vi "OOB Performance Test.vi"() -> ()   [LabVIEW 2021]
uses:
  <vilib>/Platform/TimedLoop/XDataNode/timing_clust.ctl
  <vilib>/Platform/TimedLoop/XDataNode/nitl_modes.ctl
  <vilib>/Platform/TimedLoop/XDataNode/wakeup.ctl
  CIFOutOfBand.lvclass/CIFOutOfBand.ctl
  CIFOutOfBand.lvclass
  <vilib>/Platform/TimedLoop/XDataNode/XDataNode.xnode
  <vilib>/Platform/TimedLoop/XDataNode/XDNodeRunTimeDep.lvlib
panel:
  out "avg complexwrite":dbl
  out "Max Complexwrite":dbl
  out "avg complexnote write":dbl
  out "Max Complexnote write":dbl
  out "avg complexnote":dbl
  out "Max Complexnote":dbl
  out "avg Occur":dbl
  out "Max Occur":dbl
  out "avg Notifier":dbl
  out "Max Notifier":dbl
  out "avg RTFifo":dbl
  out "Max RTFifo":dbl
  out "avg raw dvr write":dbl
  out "Max raw dvr write":dbl
  in  "stop":bool
  in  "local":cluster{"Numeric":u64}
  out "avg raw local":dbl
  out "Max raw local":dbl
  out "avg raw dvr":dbl
  out "Max raw dvr":dbl
  out "avg no conflict":dbl
  out "Max no conflict":dbl
  out "avg simple":dbl
  out "Max simple":dbl
  out "Max Complex":dbl
  out "avg complex":dbl
  out "pass":bool
  out "error out":errorcluster
  # "This test should be run on RT.  It stresses the communications by constantly creating resource contraints with the low priority sender and the high priority loop. On Windows the priority of the loops cannot be set."
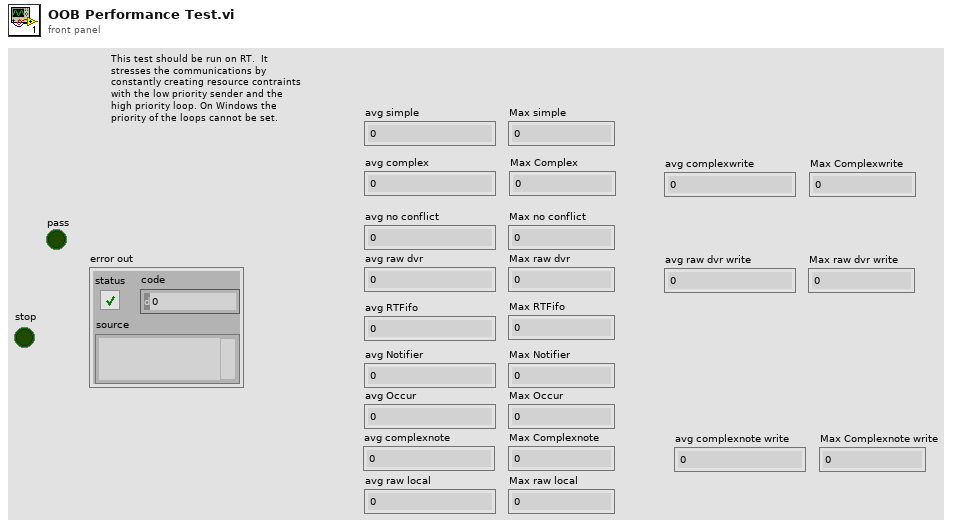
[diagram p1: front panel]
types:
  T1 = typedef "XDNodeRunTimeDep.lvlib/timing_clust.ctl" = cluster{"Expected End [f-1]":u64, "Actual End [f-1]":u64, "Finished Late? [f-1]":bool, "Expected End [i-1]":u64, "Actual End [i-1]":u64, "Finished Late? [i-1]":bool, "Expected Start [i]":u64, "Actual Start [i]":u64, "Expected Start [f]":u64, "Actual Start [f]":u64, "Source Name":string, "Structure Name":string, "Period":i64, "Deadline":i64, "Offset":i64, "Start":i64, "Priority":i32, "Timeout":i32, "Mode":T2, "Wakeup Reason":T3, "Error":errorcluster, "Source Type":string, "Secondary Source Type":string, "Global End Time":u64, "Global Start Time":u64, "Frame Duration":u64, "Iteration Duration":u64, "Assigned CPU":i32, "I/O Scan Engine Mode":u32}
  T2 = typedef "XDNodeRunTimeDep.lvlib/nitl_modes.ctl" = enum32{"No Change", "Process missed periods, maintain original phase", "Discard missed periods, maintain original phase", "Process missed periods, ignore original phase", "Discard missed periods, ignore original phase"}
  T3 = typedef "XDNodeRunTimeDep.lvlib/wakeup.ctl" = enum32{"Normal", "Aborted", "Asynchronous wakeup", "Timing source error", "Timed loop error", "Timeout"}
  T4 = cluster{"read mode":enum16{"polling", "blocking"}, "write mode":enum16{"polling", "blocking"}}
  T5 = cluster{"Numeric":dbl, "Array":cluster{"Numeric":dbl, "String":string, "Boolean":bool}[], "string":string, "Null array":u8[]}
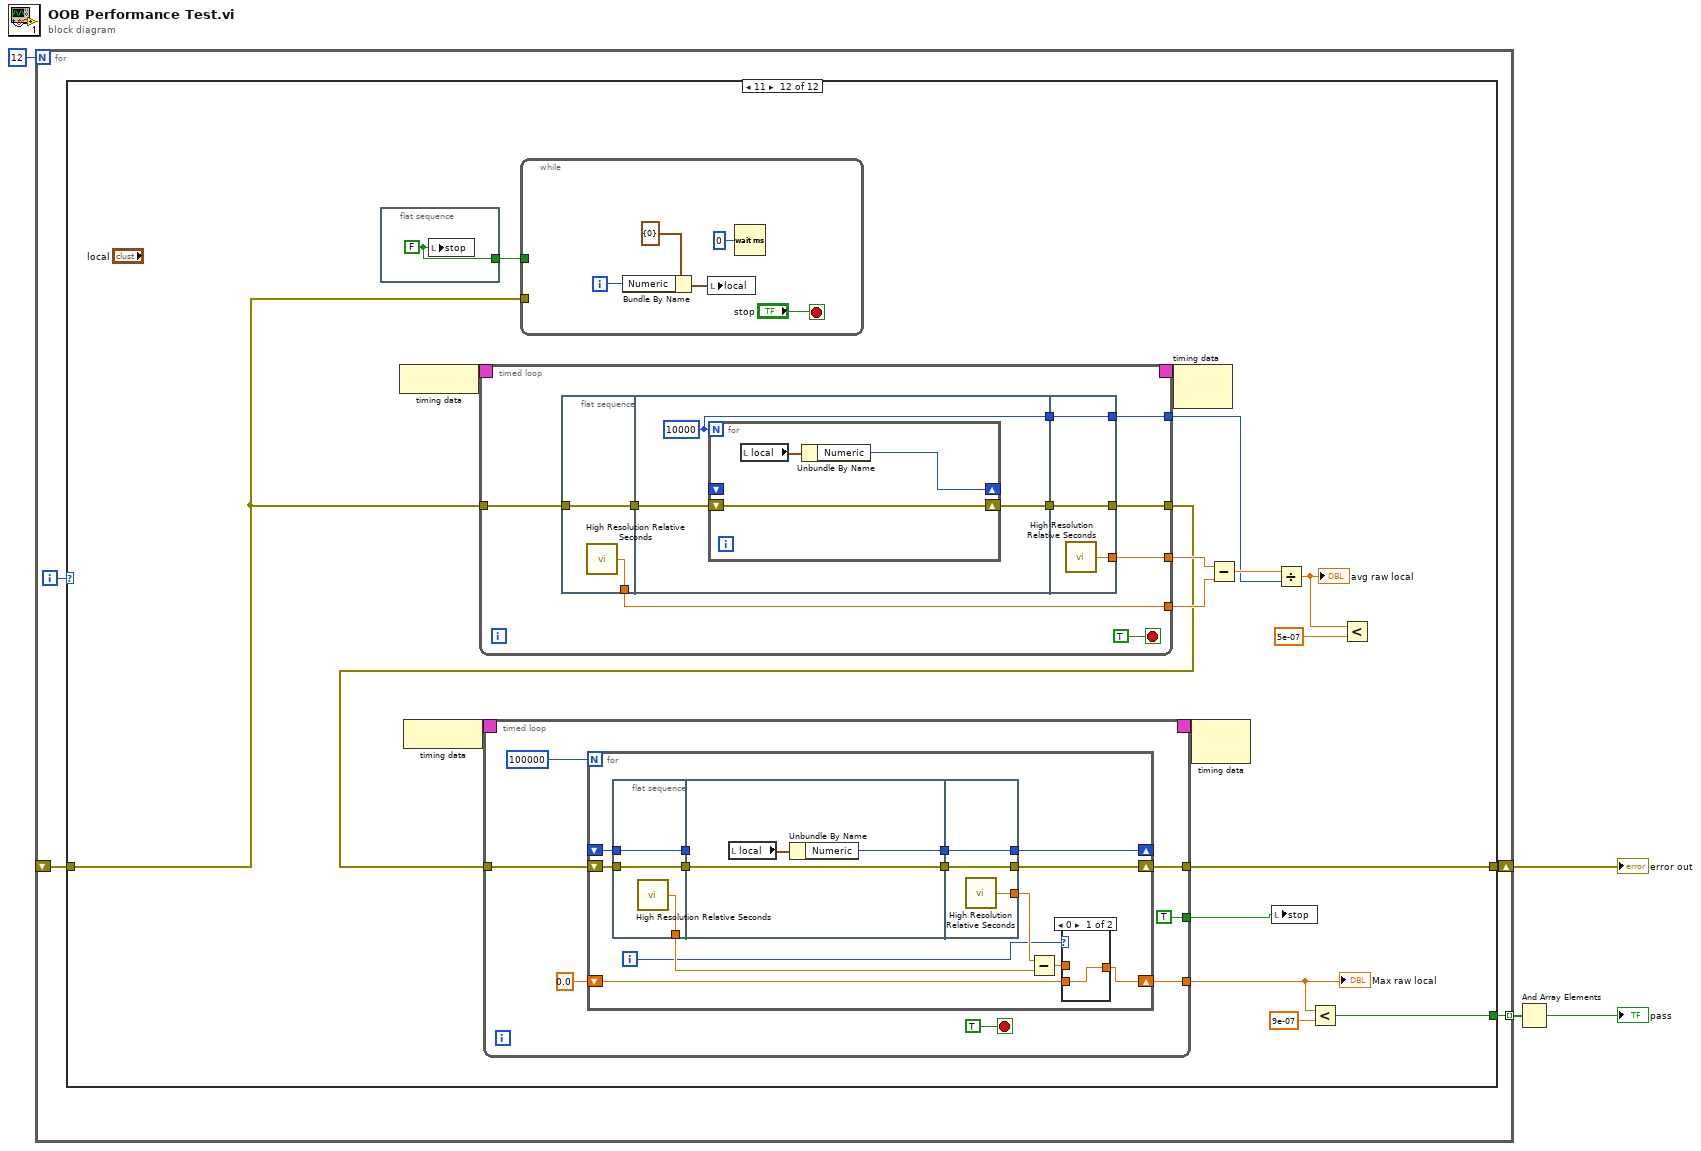
[diagram p0: block diagram]
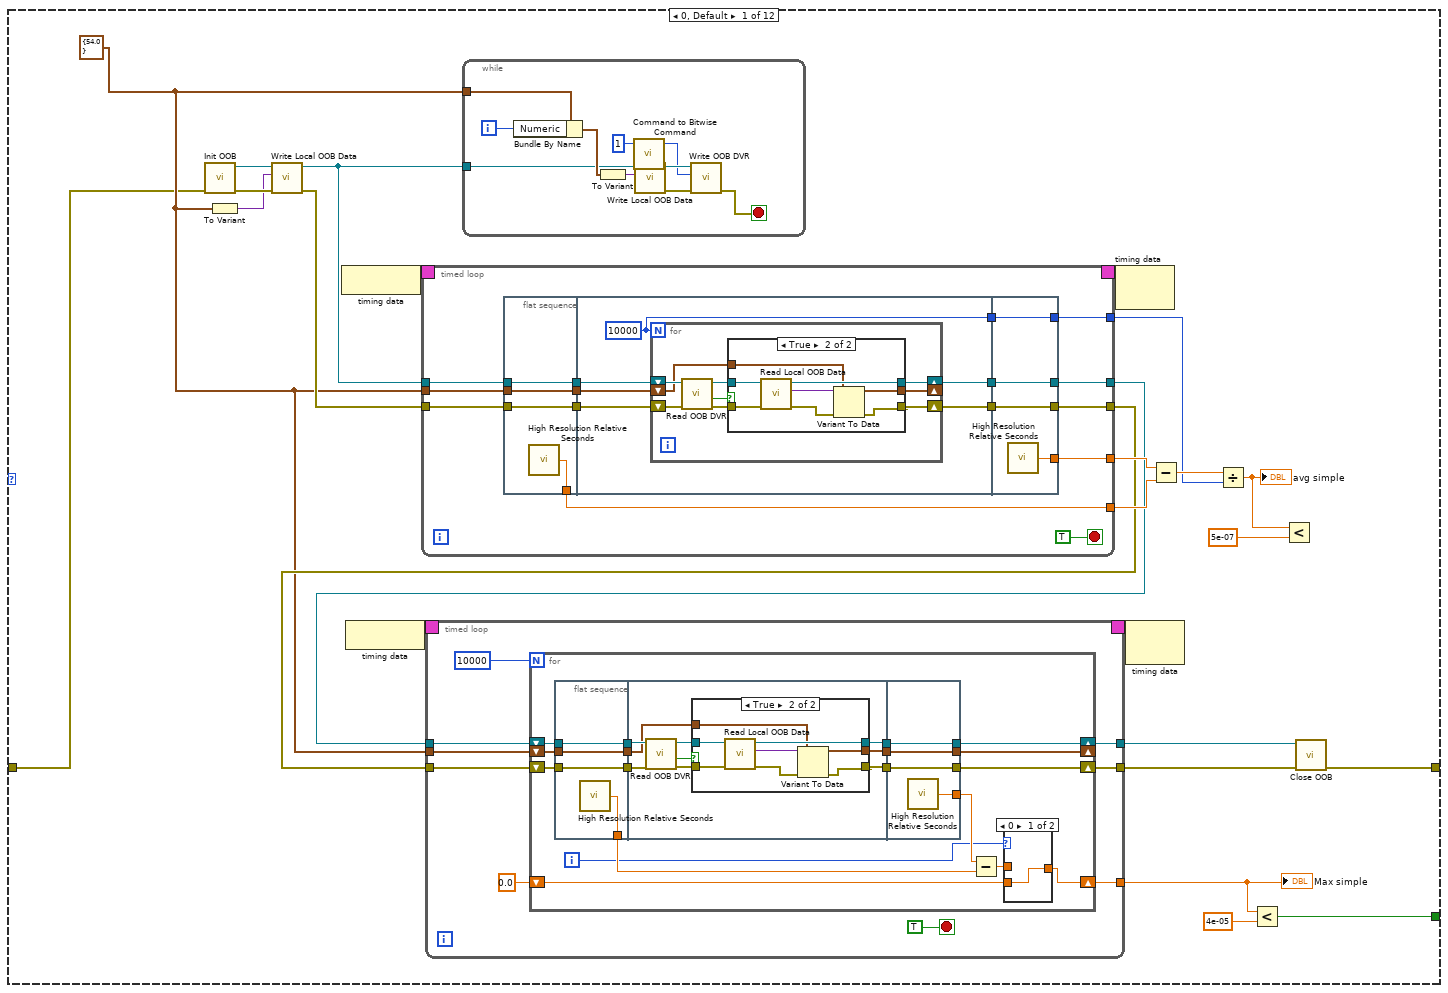
[diagram p2: hidden frame]
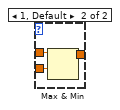
[diagram p3: hidden frame]
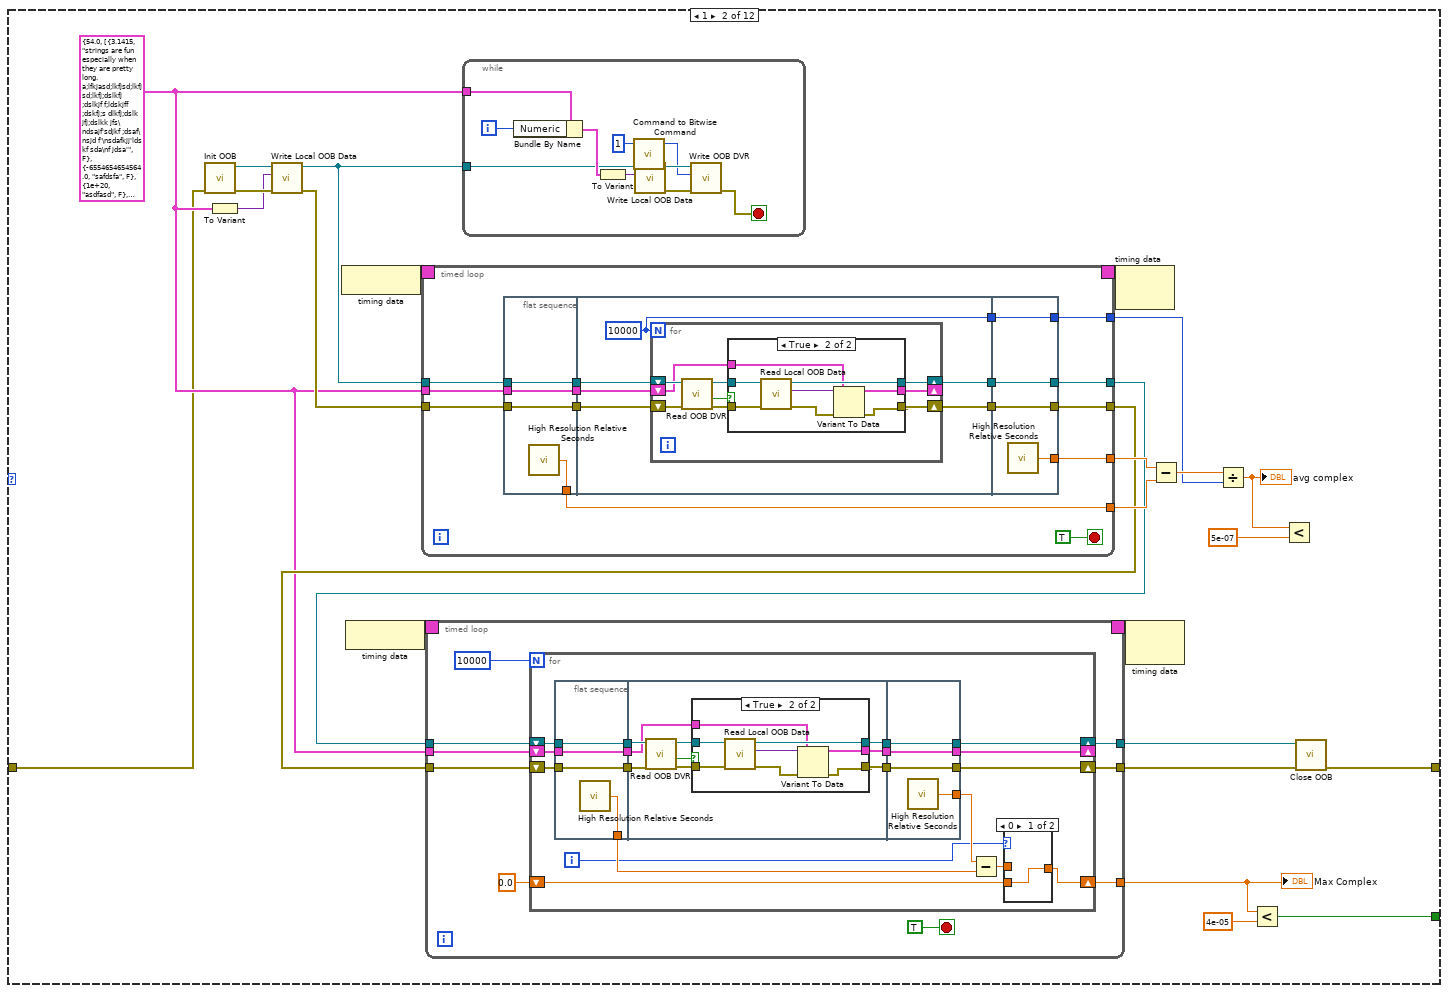
[diagram p6: hidden frame]
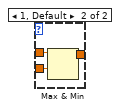
[diagram p7: hidden frame]
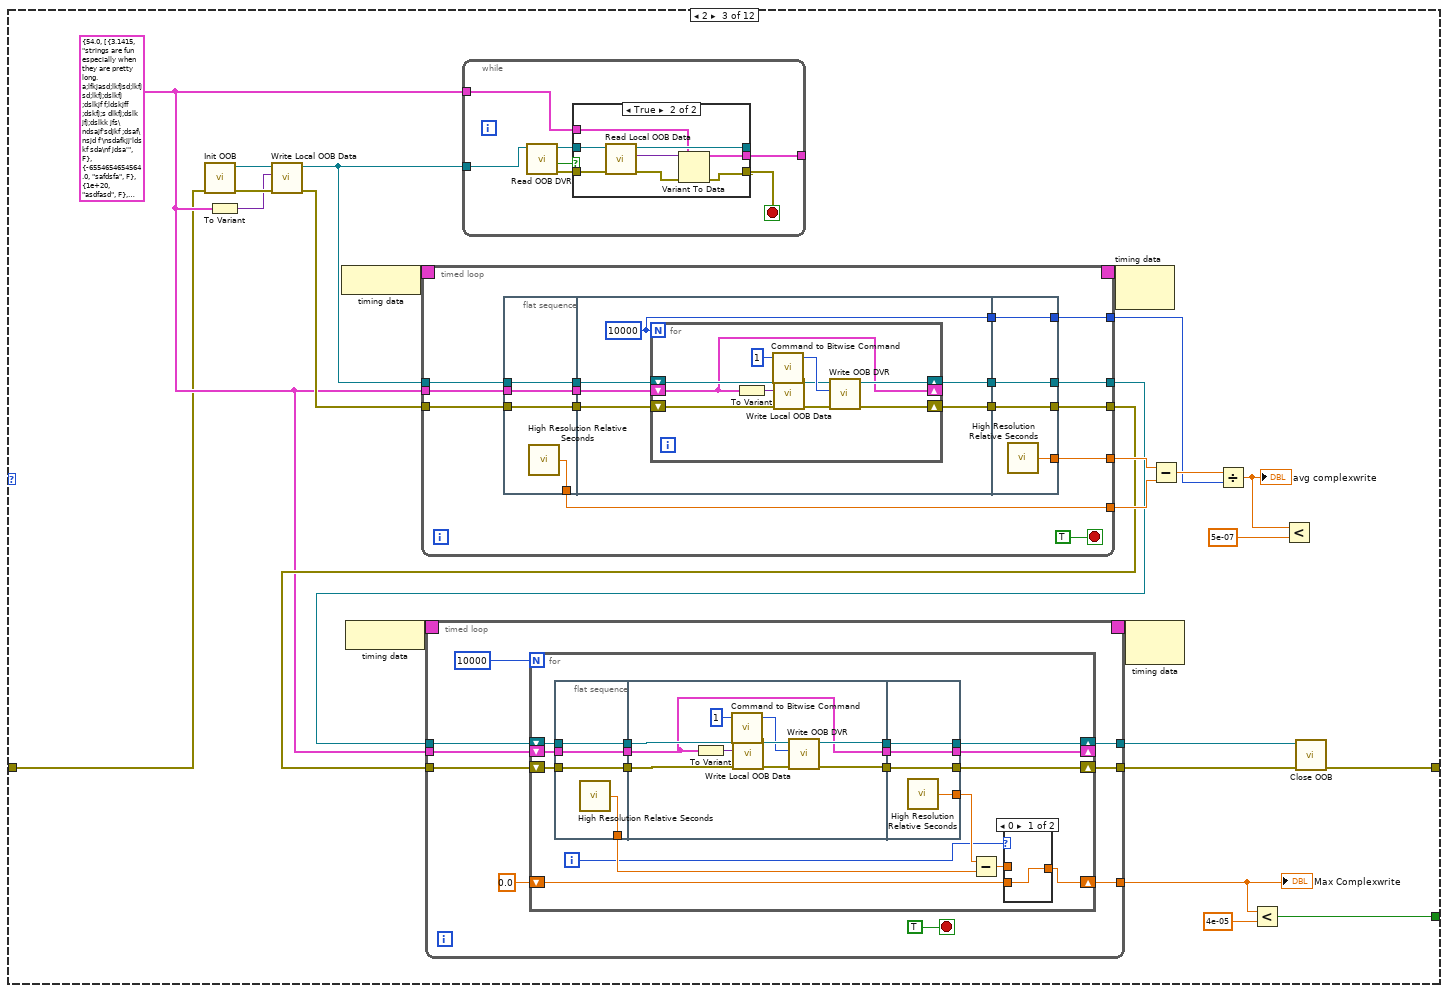
[diagram p10: hidden frame]
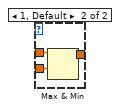
[diagram p12: hidden frame]
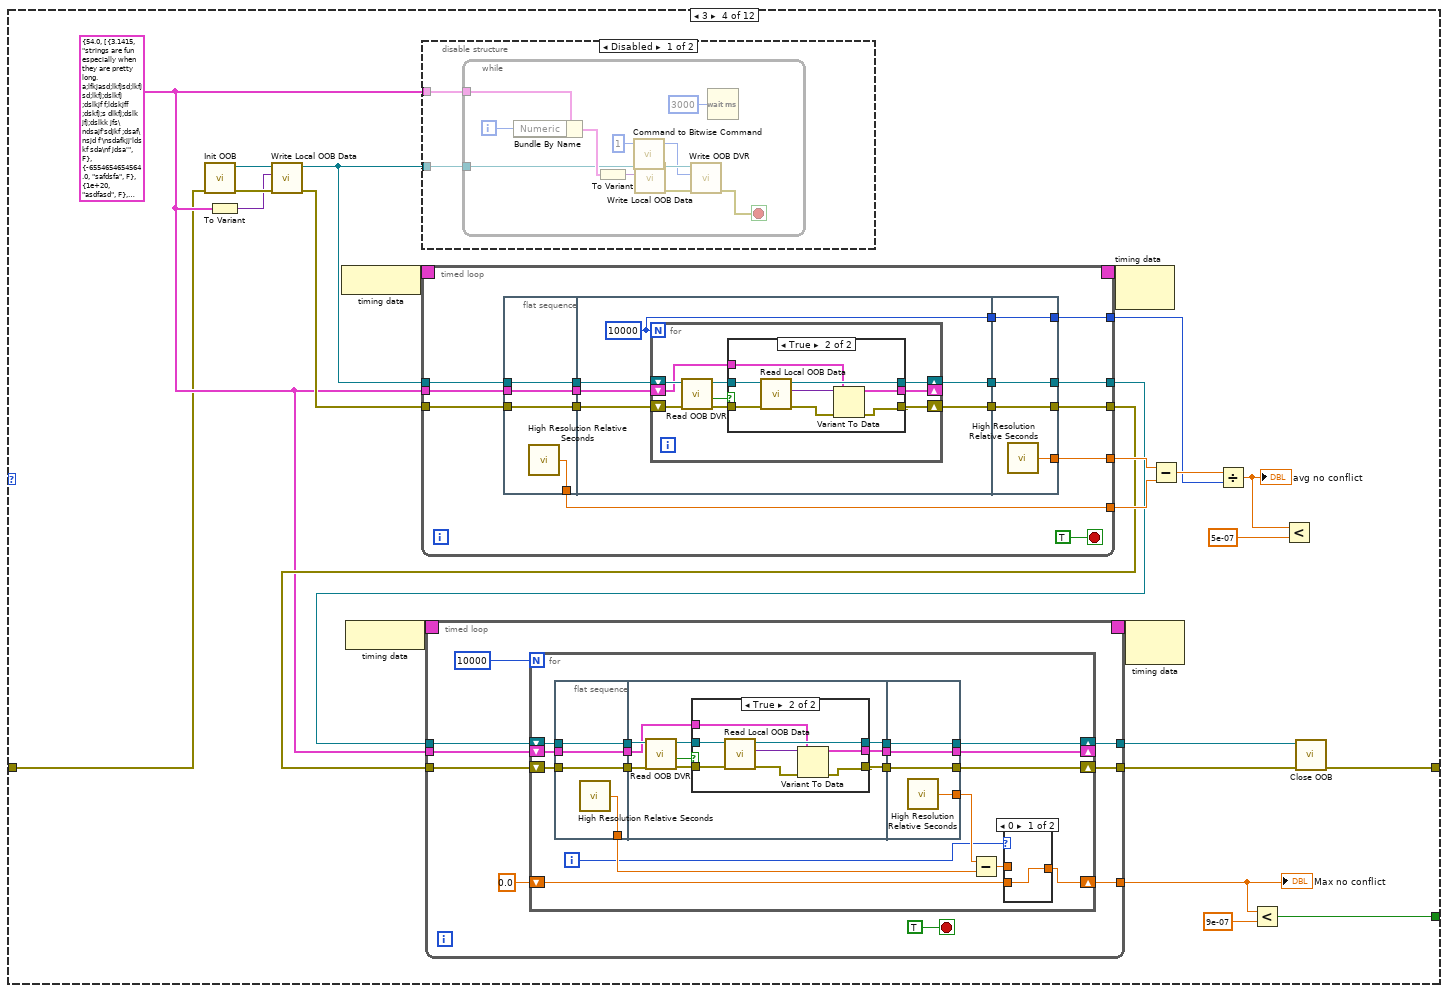
[diagram p13: hidden frame]
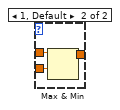
[diagram p15: hidden frame]
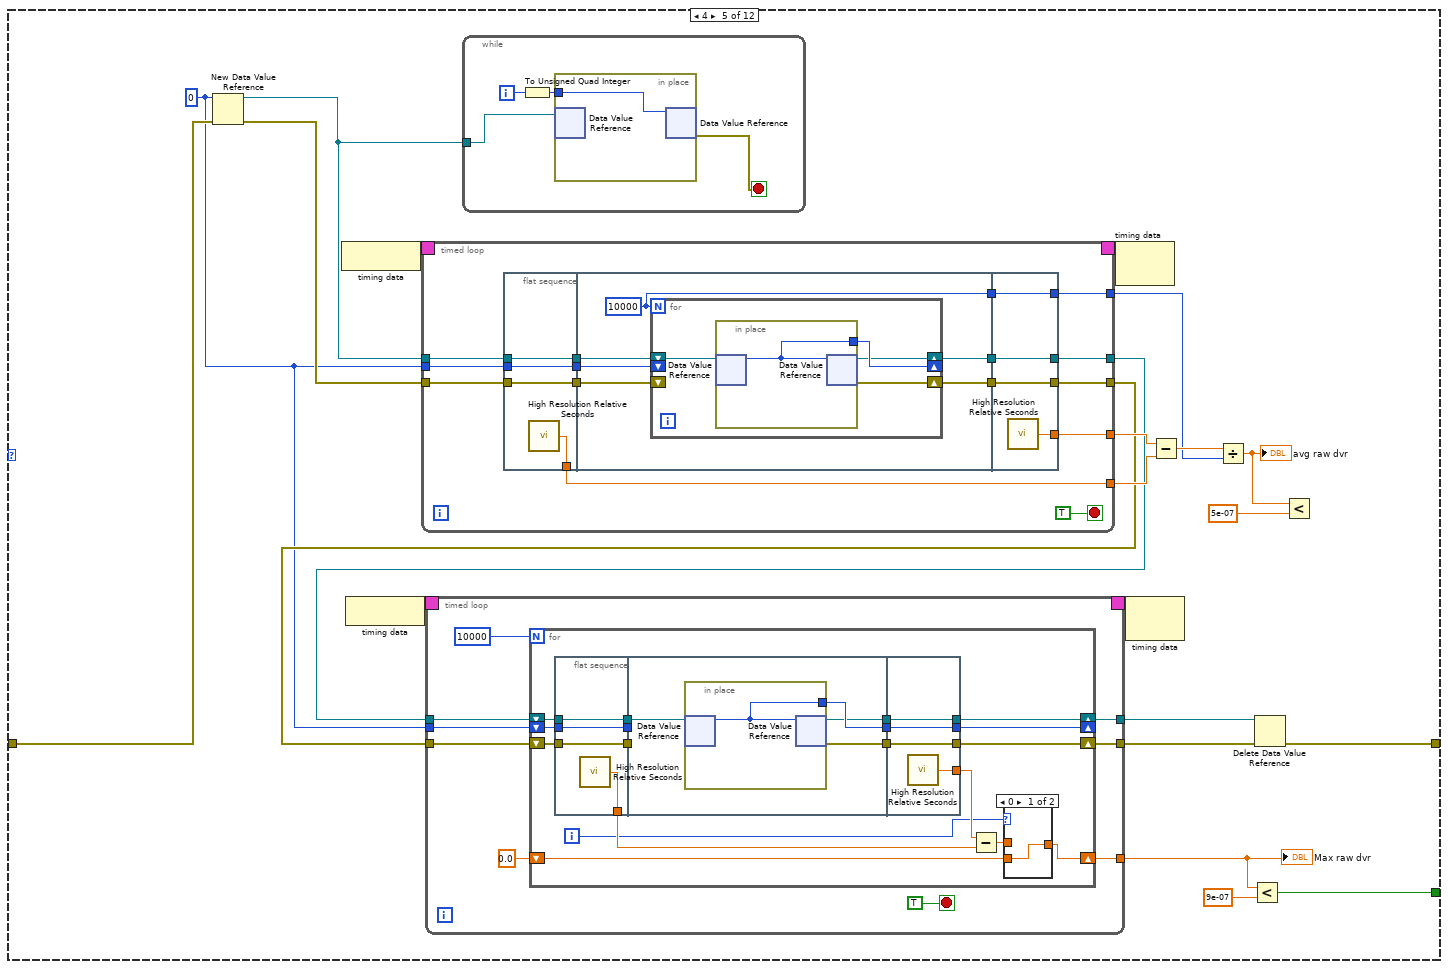
[diagram p18: hidden frame]
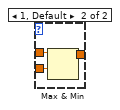
[diagram p19: hidden frame]
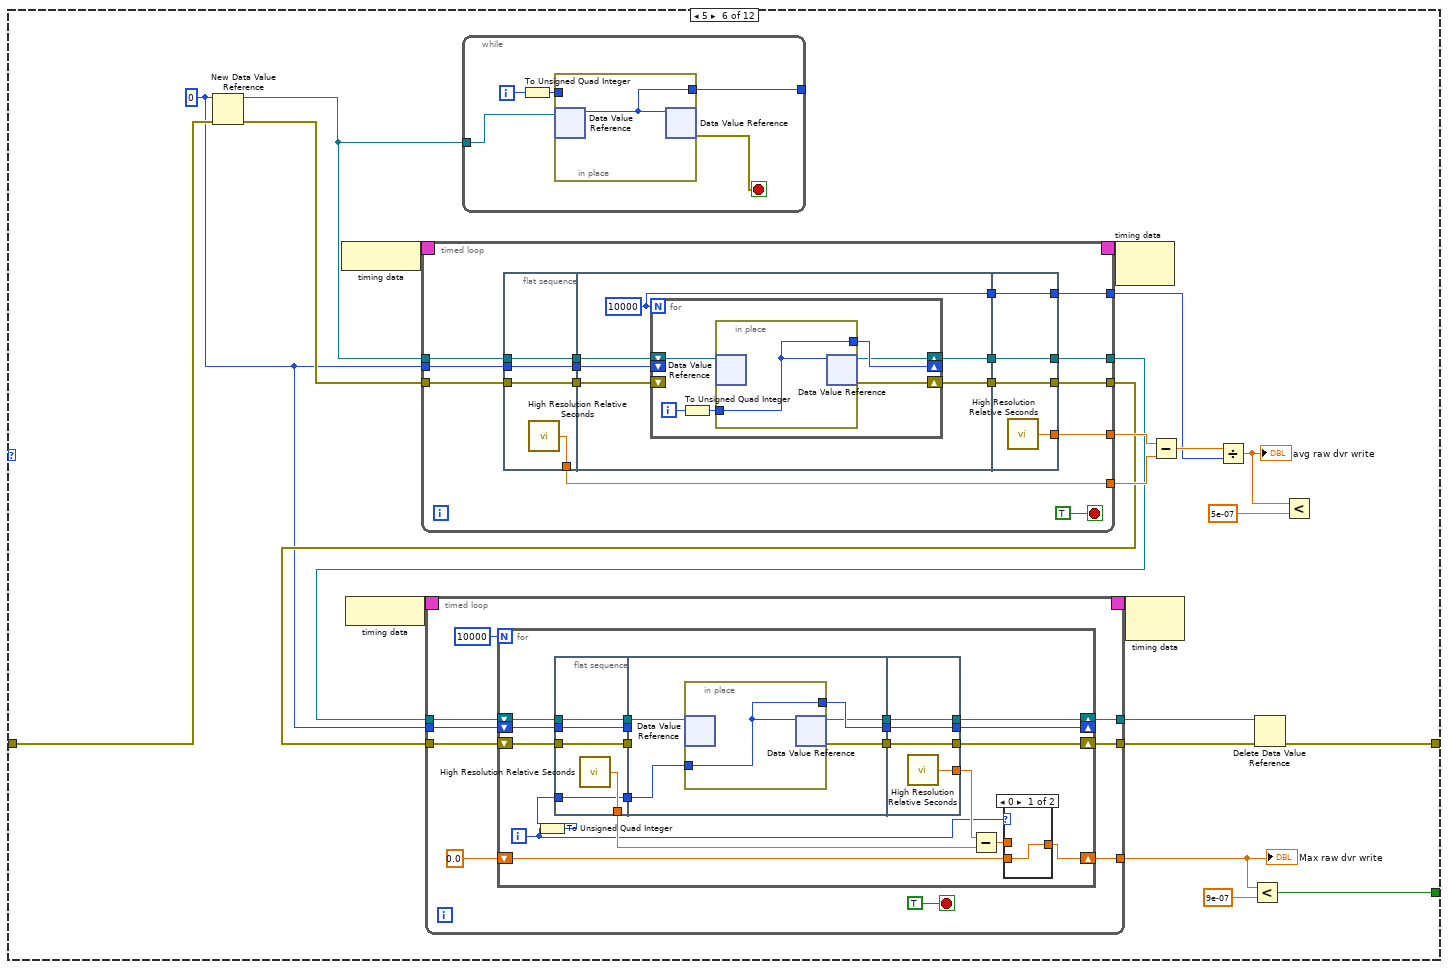
[diagram p20: hidden frame]
diagram:
  n1 = for {
    N: 12 -> [_]
    tunnel: [w8] -> w2 mode=indexing
    shift-right: [w7] -> w4
    shift-left: _ -> [w5]
    i -> [w6]
    n2 = case shown="11" w6 {
      tunnel: [w19 w168 w317 w455 w604 w717 w838 w956 w1073 w1188 w1303 w1414] -> w8
      tunnel: [w16 w165 w314 w452 w597 w710 w835 w953 w1069 w1181 w1296 w1413] -> w7
      tunnel: w5 -> [w9 w158 w307 w445 w602 w715 w832 w950 w1070 w1186 w1301 w1411]
      frame 0, Default {
        w10 = cluster{"Numeric":dbl} {"Numeric"=54.0} ("Test Config")
        n3 = call "Init OOB.vi"("error in (no error)"=w9) -> ("error out"=w15:errorcluster, "OOB out"=w13:refnum<class "CIFOutOfBand.lvclass">)  [unwired: 9 in]
        n4 = To Variant(anything=w10) -> (Variant=w14:variant)
        n5 = call "Write Local OOB Data.vi"("error in"=w15, "Local OOB Data"=w14, "OOB in"=w13) -> ("error out"=w11:errorcluster, "OOB out"=w12:refnum<class "CIFOutOfBand.lvclass">)  [unwired: 7 in]
        n6 = node-c288() -> (w33:T1)
        n7 = node-c288() -> (w31:T1)
        n8 = timed-loop {
          timing: w33 -> [_]
          timing-out: [_] -> w32
          tunnel: w12 -> [w120]
          tunnel: w11 -> [w119]
          tunnel: [w115] -> w25
          tunnel: [w113] -> w24
          tunnel: [w111] -> w29
          tunnel: [w110] -> w28
          tunnel: [w109] -> w26
          tunnel: w10 -> [w107]
          stop <- TRUE stop-if-true
          n9 = flat-sequence {
            tunnel: w119 -> [w123]
            tunnel: w120 -> [w124]
            tunnel: [w124] -> w117
            tunnel: [w123] -> w116
            tunnel: [w122] -> w110
            tunnel: w107 -> [w121]
            tunnel: [w121] -> w106
            tunnel: w117 -> [w130]
            tunnel: w116 -> [w129]
            tunnel: [w128] -> w114
            tunnel: [w127] -> w112
            tunnel: [w126] -> w108
            tunnel: w106 -> [w125]
            tunnel: [w153] -> w115
            tunnel: w114 -> [w153]
            tunnel: [w152] -> w113
            tunnel: w112 -> [w152]
            tunnel: [w151] -> w111
            tunnel: [w150] -> w109
            tunnel: w108 -> [w150]
            frame #0 {
              n10 = call <vilib>:"High Resolution Relative Seconds.vi"() -> ("relative seconds"=w122:dbl)
            }
            frame #1 {
              w126 = 10000
              n11 = for {
                N: w126 -> [_]
                shift-right: [w136] -> w128
                shift-left: w130 -> [w135]
                shift-right: [w132] -> w127
                shift-left: w129 -> [w133]
                shift-right: [w131] -> _
                shift-left: w125 -> [w134]
                n12 = call "Read OOB DVR.vi"("error in"=w133, "OOB in"=w135) -> ("error out"=w137:errorcluster, "New Commands"=w139:bool, "OOB out"=w138:refnum<class "CIFOutOfBand.lvclass">)  [unwired: 6 in, 1 out]
                n13 = case shown="True" w139 {
                  tunnel: w138 -> [w140 w149]
                  tunnel: w137 -> [w141 w148]
                  tunnel: [w140 w146] -> w136
                  tunnel: w134 -> [_ w144]
                  tunnel: [_ w142] -> w131
                  tunnel: [w141 w143] -> w132
                  frame False {
                  }
                  frame True {
                    n14 = call "Read Local OOB Data.vi"("error in"=w148, "OOB in"=w149) -> ("error out"=w147:errorcluster, "Local OOB Data"=w145:variant, "OOB out"=w146:refnum<class "CIFOutOfBand.lvclass">)  [unwired: 7 in]
                    n15 = Variant To Data(error in=w147, type=w144, Variant=w145) -> (data=w142:cluster{"Numeric":dbl}, error out=w143:errorcluster)
                  }
                }
              }
            }
            frame #2 {
              n16 = call <vilib>:"High Resolution Relative Seconds.vi"() -> ("relative seconds"=w151:dbl)
            }
          }
        }
        n17 = timed-loop {
          timing: w31 -> [_]
          timing-out: [_] -> w30
          tunnel: w25 -> [w52]
          tunnel: w24 -> [w51]
          tunnel: [w49] -> w18
          tunnel: [w48] -> w17
          tunnel: w10 -> [w47]
          tunnel: [w44] -> w21
          stop <- TRUE stop-if-true
          n18 = for {
            N: 10000 -> [_]
            shift-right: [w64] -> w49
            shift-left: w52 -> [w66]
            shift-right: [w63] -> w48
            shift-left: w51 -> [w65]
            shift-right: [w57] -> w44
            shift-left: 0.0 -> [w58]
            shift-right: [w56] -> _
            shift-left: w47 -> [w62]
            i -> [w54]
            n19 = flat-sequence {
              tunnel: w65 -> [w77]
              tunnel: w66 -> [w78]
              tunnel: [w78] -> w70
              tunnel: [w77] -> w69
              tunnel: [w76] -> w60
              tunnel: w62 -> [w75]
              tunnel: [w75] -> w68
              tunnel: w70 -> [w84]
              tunnel: w69 -> [w82]
              tunnel: [w81] -> w67
              tunnel: w68 -> [w83]
              tunnel: [w80] -> w55
              tunnel: [w79] -> w53
              tunnel: [w101] -> w64
              tunnel: w67 -> [w101]
              tunnel: [w100] -> w63
              tunnel: [w99] -> w61
              tunnel: [w98] -> w56
              tunnel: w55 -> [w98]
              tunnel: w53 -> [w100]
              frame #0 {
                n20 = call <vilib>:"High Resolution Relative Seconds.vi"() -> ("relative seconds"=w76:dbl)
              }
              frame #1 {
                n21 = call "Read OOB DVR.vi"("error in"=w82, "OOB in"=w84) -> ("error out"=w87:errorcluster, "New Commands"=w85:bool, "OOB out"=w86:refnum<class "CIFOutOfBand.lvclass">)  [unwired: 6 in, 1 out]
                n22 = case shown="True" w85 {
                  tunnel: w86 -> [w88 w97]
                  tunnel: w87 -> [w89 w96]
                  tunnel: [w88 w94] -> w81
                  tunnel: w83 -> [_ w92]
                  tunnel: [_ w90] -> w80
                  tunnel: [w89 w91] -> w79
                  frame False {
                  }
                  frame True {
                    n23 = call "Read Local OOB Data.vi"("error in"=w96, "OOB in"=w97) -> ("error out"=w95:errorcluster, "Local OOB Data"=w93:variant, "OOB out"=w94:refnum<class "CIFOutOfBand.lvclass">)  [unwired: 7 in]
                    n24 = Variant To Data(error in=w95, type=w92, Variant=w93) -> (data=w90:cluster{"Numeric":dbl}, error out=w91:errorcluster)
                  }
                }
              }
              frame #2 {
                n25 = call <vilib>:"High Resolution Relative Seconds.vi"() -> ("relative seconds"=w99:dbl)
              }
            }
            n26 = Subtract(x=w61, y=w60) -> (x-y=w59:dbl)
            n27 = case shown="0" w54 {
              tunnel: w59 -> [_ w74]
              tunnel: w58 -> [w71 w73]
              tunnel: [w71 w72] -> w57
              frame 0 {
              }
              frame 1, Default {
                n28 = Max & Min(x=w74, y=w73) -> (max(x,y)=w72:dbl)  [unwired: 1 out]
              }
            }
          }
        }
        "Max simple" <- w21
        n29 = while {
          tunnel: w12 -> [w35]
          tunnel: w10 -> [w42]
          i -> [w43]
          stop <- w34 stop-if-true
          n30 = Bundle By Name(cluster=w42, "Numeric"=w43) -> (w36:cluster{"Numeric":dbl})
          n31 = To Variant(anything=w36) -> (Variant=w38:variant)
          n32 = call "Command to Bitwise Command.vi"("OOB Command"=u8 1) -> ("bit command"=w37:u64)  [unwired: 3 in]
          n33 = call "Write Local OOB Data.vi"("Local OOB Data"=w38, "OOB in"=w35) -> ("error out"=w39:errorcluster, "OOB out"=w40:refnum<class "CIFOutOfBand.lvclass">)  [unwired: 8 in]
          n34 = call "Write OOB DVR.vi"("error in"=w39, "Commands (bitwise)"=w37, "OOB in"=w40) -> ("error out"=w34:errorcluster)  [unwired: 7 in, 1 out]
        }
        n35 = node-c288(w32) -> ()  [unwired: 1 out]
        n36 = node-c288(w30) -> ()  [unwired: 1 out]
        n37 = Subtract(x=w29, y=w28) -> (x-y=w27:dbl)
        n38 = Divide(x=w27, y=w26) -> (x/y=w23:dbl)
        "avg simple" <- w23
        n39 = Less?(x=w21, y=4e-05) -> (x < y?=w19:bool)
        n40 = Less?(x=w23, y=5e-07) -> ()  [unwired: 1 out]
        n41 = call "Close OOB.vi"("error in"=w17, "OOB in"=w18) -> ("error out"=w16:errorcluster)  [unwired: 9 in]
      }
      frame 1 {
        w159 = T5 {"Numeric"=54.0, "Array"=[{"Numeric"=3.1415, "String"="strings are fun especially when they are pretty long. a;lfkjasd;lkfjsd;lkfjsd;lkfj;dslkfj ;dslkjf f;ldskjff ;dskfj;s dlkfj;dslk jfj;dslkk jfs\ndsajf'sdjkf ;dsaf\nsjd f'\nsdafkjj'lds kf sda\nf jdsa'", "Boolean"=FALSE}, {"Numeric"=-6554654654564.0, "String"="safdsfa", "Boolean"=FALSE}, {"Numeric"=1e+20, "String"="asdfasd", "Boolean"=FALSE}, {"Numeric"=2.0, "String"="afd", "Boolean"=TRUE}, {"Numeric"=12.34, "String"="data", "Boolean"=FALSE}], "string"="strings", "Null array"=[0]} ("Test Config")
        n42 = call "Init OOB.vi"("error in (no error)"=w158) -> ("error out"=w164:errorcluster, "OOB out"=w162:refnum<class "CIFOutOfBand.lvclass">)  [unwired: 9 in]
        n43 = To Variant(anything=w159) -> (Variant=w163:variant)
        n44 = call "Write Local OOB Data.vi"("error in"=w164, "Local OOB Data"=w163, "OOB in"=w162) -> ("error out"=w160:errorcluster, "OOB out"=w161:refnum<class "CIFOutOfBand.lvclass">)  [unwired: 7 in]
        n45 = node-c288() -> (w182:T1)
        n46 = node-c288() -> (w180:T1)
        n47 = timed-loop {
          timing: w182 -> [_]
          timing-out: [_] -> w181
          tunnel: w161 -> [w269]
          tunnel: w160 -> [w268]
          tunnel: [w264] -> w174
          tunnel: [w262] -> w173
          tunnel: [w260] -> w178
          tunnel: [w259] -> w177
          tunnel: [w258] -> w175
          tunnel: w159 -> [w256]
          stop <- TRUE stop-if-true
          n48 = flat-sequence {
            tunnel: w268 -> [w272]
            tunnel: w269 -> [w273]
            tunnel: [w273] -> w266
            tunnel: [w272] -> w265
            tunnel: [w271] -> w259
            tunnel: w256 -> [w270]
            tunnel: [w270] -> w255
            tunnel: w266 -> [w279]
            tunnel: w265 -> [w278]
            tunnel: [w277] -> w263
            tunnel: [w276] -> w261
            tunnel: [w275] -> w257
            tunnel: w255 -> [w274]
            tunnel: [w302] -> w264
            tunnel: w263 -> [w302]
            tunnel: [w301] -> w262
            tunnel: w261 -> [w301]
            tunnel: [w300] -> w260
            tunnel: [w299] -> w258
            tunnel: w257 -> [w299]
            frame #0 {
              n49 = call <vilib>:"High Resolution Relative Seconds.vi"() -> ("relative seconds"=w271:dbl)
            }
            frame #1 {
              w275 = 10000
              n50 = for {
                N: w275 -> [_]
                shift-right: [w285] -> w277
                shift-left: w279 -> [w284]
                shift-right: [w281] -> w276
                shift-left: w278 -> [w282]
                shift-right: [w280] -> _
                shift-left: w274 -> [w283]
                n51 = call "Read OOB DVR.vi"("error in"=w282, "OOB in"=w284) -> ("error out"=w286:errorcluster, "New Commands"=w288:bool, "OOB out"=w287:refnum<class "CIFOutOfBand.lvclass">)  [unwired: 6 in, 1 out]
                n52 = case shown="True" w288 {
                  tunnel: w287 -> [w289 w298]
                  tunnel: w286 -> [w290 w297]
                  tunnel: [w289 w295] -> w285
                  tunnel: w283 -> [_ w293]
                  tunnel: [_ w291] -> w280
                  tunnel: [w290 w292] -> w281
                  frame False {
                  }
                  frame True {
                    n53 = call "Read Local OOB Data.vi"("error in"=w297, "OOB in"=w298) -> ("error out"=w296:errorcluster, "Local OOB Data"=w294:variant, "OOB out"=w295:refnum<class "CIFOutOfBand.lvclass">)  [unwired: 7 in]
                    n54 = Variant To Data(error in=w296, type=w293, Variant=w294) -> (data=w291:T5, error out=w292:errorcluster)
                  }
                }
              }
            }
            frame #2 {
              n55 = call <vilib>:"High Resolution Relative Seconds.vi"() -> ("relative seconds"=w300:dbl)
            }
          }
        }
        n56 = timed-loop {
          timing: w180 -> [_]
          timing-out: [_] -> w179
          tunnel: w174 -> [w201]
          tunnel: w173 -> [w200]
          tunnel: [w198] -> w167
          tunnel: [w197] -> w166
          tunnel: w159 -> [w196]
          tunnel: [w193] -> w170
          stop <- TRUE stop-if-true
          n57 = for {
            N: 10000 -> [_]
            shift-right: [w213] -> w198
            shift-left: w201 -> [w215]
            shift-right: [w212] -> w197
            shift-left: w200 -> [w214]
            shift-right: [w206] -> w193
            shift-left: 0.0 -> [w207]
            shift-right: [w205] -> _
            shift-left: w196 -> [w211]
            i -> [w203]
            n58 = flat-sequence {
              tunnel: w214 -> [w226]
              tunnel: w215 -> [w227]
              tunnel: [w227] -> w219
              tunnel: [w226] -> w218
              tunnel: [w225] -> w209
              tunnel: w211 -> [w224]
              tunnel: [w224] -> w217
              tunnel: w219 -> [w233]
              tunnel: w218 -> [w231]
              tunnel: [w230] -> w216
              tunnel: w217 -> [w232]
              tunnel: [w229] -> w204
              tunnel: [w228] -> w202
              tunnel: [w250] -> w213
              tunnel: w216 -> [w250]
              tunnel: [w249] -> w212
              tunnel: [w248] -> w210
              tunnel: [w247] -> w205
              tunnel: w204 -> [w247]
              tunnel: w202 -> [w249]
              frame #0 {
                n59 = call <vilib>:"High Resolution Relative Seconds.vi"() -> ("relative seconds"=w225:dbl)
              }
              frame #1 {
                n60 = call "Read OOB DVR.vi"("error in"=w231, "OOB in"=w233) -> ("error out"=w236:errorcluster, "New Commands"=w234:bool, "OOB out"=w235:refnum<class "CIFOutOfBand.lvclass">)  [unwired: 6 in, 1 out]
                n61 = case shown="True" w234 {
                  tunnel: w235 -> [w237 w246]
                  tunnel: w236 -> [w238 w245]
                  tunnel: [w237 w243] -> w230
                  tunnel: w232 -> [_ w241]
                  tunnel: [_ w239] -> w229
                  tunnel: [w238 w240] -> w228
                  frame False {
                  }
                  frame True {
                    n62 = call "Read Local OOB Data.vi"("error in"=w245, "OOB in"=w246) -> ("error out"=w244:errorcluster, "Local OOB Data"=w242:variant, "OOB out"=w243:refnum<class "CIFOutOfBand.lvclass">)  [unwired: 7 in]
                    n63 = Variant To Data(error in=w244, type=w241, Variant=w242) -> (data=w239:T5, error out=w240:errorcluster)
                  }
                }
              }
              frame #2 {
                n64 = call <vilib>:"High Resolution Relative Seconds.vi"() -> ("relative seconds"=w248:dbl)
              }
            }
            n65 = Subtract(x=w210, y=w209) -> (x-y=w208:dbl)
            n66 = case shown="0" w203 {
              tunnel: w208 -> [_ w223]
              tunnel: w207 -> [w220 w222]
              tunnel: [w220 w221] -> w206
              frame 0 {
              }
              frame 1, Default {
                n67 = Max & Min(x=w223, y=w222) -> (max(x,y)=w221:dbl)  [unwired: 1 out]
              }
            }
          }
        }
        "Max Complex" <- w170
        n68 = while {
          tunnel: w161 -> [w184]
          tunnel: w159 -> [w191]
          i -> [w192]
          stop <- w183 stop-if-true
          n69 = Bundle By Name(cluster=w191, "Numeric"=w192) -> (w185:T5)
          n70 = To Variant(anything=w185) -> (Variant=w187:variant)
          n71 = call "Command to Bitwise Command.vi"("OOB Command"=u8 1) -> ("bit command"=w186:u64)  [unwired: 3 in]
          n72 = call "Write Local OOB Data.vi"("Local OOB Data"=w187, "OOB in"=w184) -> ("error out"=w188:errorcluster, "OOB out"=w189:refnum<class "CIFOutOfBand.lvclass">)  [unwired: 8 in]
          n73 = call "Write OOB DVR.vi"("error in"=w188, "Commands (bitwise)"=w186, "OOB in"=w189) -> ("error out"=w183:errorcluster)  [unwired: 7 in, 1 out]
        }
        n74 = node-c288(w181) -> ()  [unwired: 1 out]
        n75 = node-c288(w179) -> ()  [unwired: 1 out]
        n76 = Subtract(x=w178, y=w177) -> (x-y=w176:dbl)
        n77 = Divide(x=w176, y=w175) -> (x/y=w172:dbl)
        "avg complex" <- w172
        n78 = Less?(x=w170, y=4e-05) -> (x < y?=w168:bool)
        n79 = Less?(x=w172, y=5e-07) -> ()  [unwired: 1 out]
        n80 = call "Close OOB.vi"("error in"=w166, "OOB in"=w167) -> ("error out"=w165:errorcluster)  [unwired: 9 in]
      }
      frame 2 {
        w308 = T5 {"Numeric"=54.0, "Array"=[{"Numeric"=3.1415, "String"="strings are fun especially when they are pretty long. a;lfkjasd;lkfjsd;lkfjsd;lkfj;dslkfj ;dslkjf f;ldskjff ;dskfj;s dlkfj;dslk jfj;dslkk jfs\ndsajf'sdjkf ;dsaf\nsjd f'\nsdafkjj'lds kf sda\nf jdsa'", "Boolean"=FALSE}, {"Numeric"=-6554654654564.0, "String"="safdsfa", "Boolean"=FALSE}, {"Numeric"=1e+20, "String"="asdfasd", "Boolean"=FALSE}, {"Numeric"=2.0, "String"="afd", "Boolean"=TRUE}, {"Numeric"=12.34, "String"="data", "Boolean"=FALSE}], "string"="strings", "Null array"=[0]} ("Test Config")
        n81 = call "Init OOB.vi"("error in (no error)"=w307) -> ("error out"=w313:errorcluster, "OOB out"=w311:refnum<class "CIFOutOfBand.lvclass">)  [unwired: 9 in]
        n82 = To Variant(anything=w308) -> (Variant=w312:variant)
        n83 = call "Write Local OOB Data.vi"("error in"=w313, "Local OOB Data"=w312, "OOB in"=w311) -> ("error out"=w309:errorcluster, "OOB out"=w310:refnum<class "CIFOutOfBand.lvclass">)  [unwired: 7 in]
        n84 = node-c288() -> (w331:T1)
        n85 = node-c288() -> (w329:T1)
        n86 = timed-loop {
          timing: w331 -> [_]
          timing-out: [_] -> w330
          tunnel: w310 -> [w416]
          tunnel: w309 -> [w415]
          tunnel: [w411] -> w323
          tunnel: [w409] -> w322
          tunnel: [w407] -> w327
          tunnel: [w406] -> w326
          tunnel: [w405] -> w324
          tunnel: w308 -> [w403]
          stop <- TRUE stop-if-true
          n87 = flat-sequence {
            tunnel: w415 -> [w419]
            tunnel: w416 -> [w420]
            tunnel: [w420] -> w413
            tunnel: [w419] -> w412
            tunnel: [w418] -> w406
            tunnel: w403 -> [w417]
            tunnel: [w417] -> w402
            tunnel: w413 -> [w426]
            tunnel: w412 -> [w425]
            tunnel: [w424] -> w410
            tunnel: [w423] -> w408
            tunnel: [w422] -> w404
            tunnel: w402 -> [w421]
            tunnel: [w440] -> w411
            tunnel: w410 -> [w440]
            tunnel: [w439] -> w409
            tunnel: w408 -> [w439]
            tunnel: [w438] -> w407
            tunnel: [w437] -> w405
            tunnel: w404 -> [w437]
            frame #0 {
              n88 = call <vilib>:"High Resolution Relative Seconds.vi"() -> ("relative seconds"=w418:dbl)
            }
            frame #1 {
              w422 = 10000
              n89 = for {
                N: w422 -> [_]
                shift-right: [w428] -> w424
                shift-left: w426 -> [w429]
                shift-right: [w430] -> w423
                shift-left: w425 -> [w431]
                shift-right: [w427] -> _
                shift-left: w421 -> [w427]
                n90 = To Variant(anything=w427) -> (Variant=w435:variant)
                n91 = call "Command to Bitwise Command.vi"("OOB Command"=u8 1) -> ("bit command"=w436:u64)  [unwired: 3 in]
                n92 = call "Write Local OOB Data.vi"("error in"=w431, "Local OOB Data"=w435, "OOB in"=w429) -> ("error out"=w434:errorcluster, "OOB out"=w433:refnum<class "CIFOutOfBand.lvclass">)  [unwired: 7 in]
                n93 = call "Write OOB DVR.vi"("error in"=w434, "Commands (bitwise)"=w436, "OOB in"=w433) -> ("error out"=w430:errorcluster, "OOB out"=w428:refnum<class "CIFOutOfBand.lvclass">)  [unwired: 7 in]
              }
            }
            frame #2 {
              n94 = call <vilib>:"High Resolution Relative Seconds.vi"() -> ("relative seconds"=w438:dbl)
            }
          }
        }
        n95 = timed-loop {
          timing: w329 -> [_]
          timing-out: [_] -> w328
          tunnel: w323 -> [w357]
          tunnel: w322 -> [w356]
          tunnel: [w354] -> w316
          tunnel: [w353] -> w315
          tunnel: w308 -> [w352]
          tunnel: [w349] -> w319
          stop <- TRUE stop-if-true
          n96 = for {
            N: 10000 -> [_]
            shift-right: [w369] -> w354
            shift-left: w357 -> [w371]
            shift-right: [w368] -> w353
            shift-left: w356 -> [w370]
            shift-right: [w362] -> w349
            shift-left: 0.0 -> [w363]
            shift-right: [w361] -> _
            shift-left: w352 -> [w367]
            i -> [w360]
            n97 = flat-sequence {
              tunnel: w370 -> [w382]
              tunnel: w371 -> [w383]
              tunnel: [w383] -> w375
              tunnel: [w382] -> w374
              tunnel: [w381] -> w365
              tunnel: w367 -> [w380]
              tunnel: [w380] -> w373
              tunnel: w375 -> [w387]
              tunnel: w374 -> [w388]
              tunnel: [w385] -> w372
              tunnel: w373 -> [w384]
              tunnel: [w386] -> w359
              tunnel: [w384] -> w358
              tunnel: [w397] -> w369
              tunnel: w372 -> [w397]
              tunnel: [w396] -> w368
              tunnel: [w395] -> w366
              tunnel: [w394] -> w361
              tunnel: w359 -> [w396]
              tunnel: w358 -> [w394]
              frame #0 {
                n98 = call <vilib>:"High Resolution Relative Seconds.vi"() -> ("relative seconds"=w381:dbl)
              }
              frame #1 {
                n99 = To Variant(anything=w384) -> (Variant=w390:variant)
                n100 = call "Command to Bitwise Command.vi"("OOB Command"=u8 1) -> ("bit command"=w389:u64)  [unwired: 3 in]
                n101 = call "Write Local OOB Data.vi"("error in"=w388, "Local OOB Data"=w390, "OOB in"=w387) -> ("error out"=w391:errorcluster, "OOB out"=w392:refnum<class "CIFOutOfBand.lvclass">)  [unwired: 7 in]
                n102 = call "Write OOB DVR.vi"("error in"=w391, "Commands (bitwise)"=w389, "OOB in"=w392) -> ("error out"=w386:errorcluster, "OOB out"=w385:refnum<class "CIFOutOfBand.lvclass">)  [unwired: 7 in]
              }
              frame #2 {
                n103 = call <vilib>:"High Resolution Relative Seconds.vi"() -> ("relative seconds"=w395:dbl)
              }
            }
            n104 = Subtract(x=w366, y=w365) -> (x-y=w364:dbl)
            n105 = case shown="0" w360 {
              tunnel: w364 -> [_ w379]
              tunnel: w363 -> [w376 w378]
              tunnel: [w376 w377] -> w362
              frame 0 {
              }
              frame 1, Default {
                n106 = Max & Min(x=w379, y=w378) -> (max(x,y)=w377:dbl)  [unwired: 1 out]
              }
            }
          }
        }
        "Max Complexwrite" <- w319
        n107 = while {
          tunnel: w310 -> [w333]
          tunnel: w308 -> [w334]
          tunnel: [w332] -> _
          stop <- w335 stop-if-true
          n108 = call "Read OOB DVR.vi"("OOB in"=w333) -> ("error out"=w336:errorcluster, "New Commands"=w338:bool, "OOB out"=w337:refnum<class "CIFOutOfBand.lvclass">)  [unwired: 7 in, 1 out]
          n109 = case shown="True" w338 {
            tunnel: w337 -> [w339 w348]
            tunnel: w336 -> [w340 w347]
            tunnel: [w339 w345] -> _
            tunnel: w334 -> [_ w343]
            tunnel: [_ w341] -> w332
            tunnel: [w340 w342] -> w335
            frame False {
            }
            frame True {
              n110 = call "Read Local OOB Data.vi"("error in"=w347, "OOB in"=w348) -> ("error out"=w346:errorcluster, "Local OOB Data"=w344:variant, "OOB out"=w345:refnum<class "CIFOutOfBand.lvclass">)  [unwired: 7 in]
              n111 = Variant To Data(error in=w346, type=w343, Variant=w344) -> (data=w341:T5, error out=w342:errorcluster)
            }
          }
        }
        n112 = node-c288(w330) -> ()  [unwired: 1 out]
        n113 = node-c288(w328) -> ()  [unwired: 1 out]
        n114 = Subtract(x=w327, y=w326) -> (x-y=w325:dbl)
        n115 = Divide(x=w325, y=w324) -> (x/y=w321:dbl)
        "avg complexwrite" <- w321
        n116 = Less?(x=w319, y=4e-05) -> (x < y?=w317:bool)
        n117 = Less?(x=w321, y=5e-07) -> ()  [unwired: 1 out]
        n118 = call "Close OOB.vi"("error in"=w315, "OOB in"=w316) -> ("error out"=w314:errorcluster)  [unwired: 9 in]
      }
      frame 3 {
        w446 = T5 {"Numeric"=54.0, "Array"=[{"Numeric"=3.1415, "String"="strings are fun especially when they are pretty long. a;lfkjasd;lkfjsd;lkfjsd;lkfj;dslkfj ;dslkjf f;ldskjff ;dskfj;s dlkfj;dslk jfj;dslkk jfs\ndsajf'sdjkf ;dsaf\nsjd f'\nsdafkjj'lds kf sda\nf jdsa'", "Boolean"=FALSE}, {"Numeric"=-6554654654564.0, "String"="safdsfa", "Boolean"=FALSE}, {"Numeric"=1e+20, "String"="asdfasd", "Boolean"=FALSE}, {"Numeric"=2.0, "String"="afd", "Boolean"=TRUE}, {"Numeric"=12.34, "String"="data", "Boolean"=FALSE}], "string"="strings", "Null array"=[0]} ("Test Config")
        n119 = call "Init OOB.vi"("error in (no error)"=w445) -> ("error out"=w451:errorcluster, "OOB out"=w449:refnum<class "CIFOutOfBand.lvclass">)  [unwired: 9 in]
        n120 = To Variant(anything=w446) -> (Variant=w450:variant)
        n121 = call "Write Local OOB Data.vi"("error in"=w451, "Local OOB Data"=w450, "OOB in"=w449) -> ("error out"=w447:errorcluster, "OOB out"=w448:refnum<class "CIFOutOfBand.lvclass">)  [unwired: 7 in]
        n122 = node-c288() -> (w469:T1)
        n123 = node-c288() -> (w467:T1)
        n124 = timed-loop {
          timing: w469 -> [_]
          timing-out: [_] -> w468
          tunnel: w448 -> [w559]
          tunnel: w447 -> [w558]
          tunnel: [w554] -> w461
          tunnel: [w552] -> w460
          tunnel: [w550] -> w465
          tunnel: [w549] -> w464
          tunnel: [w548] -> w462
          tunnel: w446 -> [w546]
          stop <- TRUE stop-if-true
          n125 = flat-sequence {
            tunnel: w558 -> [w562]
            tunnel: w559 -> [w563]
            tunnel: [w563] -> w556
            tunnel: [w562] -> w555
            tunnel: [w561] -> w549
            tunnel: w546 -> [w560]
            tunnel: [w560] -> w545
            tunnel: w556 -> [w569]
            tunnel: w555 -> [w568]
            tunnel: [w567] -> w553
            tunnel: [w566] -> w551
            tunnel: [w565] -> w547
            tunnel: w545 -> [w564]
            tunnel: [w592] -> w554
            tunnel: w553 -> [w592]
            tunnel: [w591] -> w552
            tunnel: w551 -> [w591]
            tunnel: [w590] -> w550
            tunnel: [w589] -> w548
            tunnel: w547 -> [w589]
            frame #0 {
              n126 = call <vilib>:"High Resolution Relative Seconds.vi"() -> ("relative seconds"=w561:dbl)
            }
            frame #1 {
              w565 = 10000
              n127 = for {
                N: w565 -> [_]
                shift-right: [w575] -> w567
                shift-left: w569 -> [w574]
                shift-right: [w571] -> w566
                shift-left: w568 -> [w572]
                shift-right: [w570] -> _
                shift-left: w564 -> [w573]
                n128 = call "Read OOB DVR.vi"("error in"=w572, "OOB in"=w574) -> ("error out"=w576:errorcluster, "New Commands"=w578:bool, "OOB out"=w577:refnum<class "CIFOutOfBand.lvclass">)  [unwired: 6 in, 1 out]
                n129 = case shown="True" w578 {
                  tunnel: w577 -> [w579 w588]
                  tunnel: w576 -> [w580 w587]
                  tunnel: [w579 w585] -> w575
                  tunnel: w573 -> [_ w583]
                  tunnel: [_ w581] -> w570
                  tunnel: [w580 w582] -> w571
                  frame False {
                  }
                  frame True {
                    n130 = call "Read Local OOB Data.vi"("error in"=w587, "OOB in"=w588) -> ("error out"=w586:errorcluster, "Local OOB Data"=w584:variant, "OOB out"=w585:refnum<class "CIFOutOfBand.lvclass">)  [unwired: 7 in]
                    n131 = Variant To Data(error in=w586, type=w583, Variant=w584) -> (data=w581:T5, error out=w582:errorcluster)
                  }
                }
              }
            }
            frame #2 {
              n132 = call <vilib>:"High Resolution Relative Seconds.vi"() -> ("relative seconds"=w590:dbl)
            }
          }
        }
        n133 = disable-structure shown="Disabled" {
          disable-tunnel: w448 -> [w471 _]
          disable-tunnel: w446 -> [w470 _]
          frame Disabled {
            n134 = while {
              tunnel: w471 -> [w474]
              tunnel: w470 -> [w481]
              i -> [w482]
              stop <- w473 stop-if-true
              n135 = Bundle By Name(cluster=w481, "Numeric"=w482) -> (w475:T5)
              n136 = To Variant(anything=w475) -> (Variant=w477:variant)
              n137 = call "Command to Bitwise Command.vi"("OOB Command"=u8 1) -> ("bit command"=w476:u64)  [unwired: 3 in]
              n138 = call "Write Local OOB Data.vi"("Local OOB Data"=w477, "OOB in"=w474) -> ("error out"=w478:errorcluster, "OOB out"=w479:refnum<class "CIFOutOfBand.lvclass">)  [unwired: 8 in]
              n139 = call "Write OOB DVR.vi"("error in"=w478, "Commands (bitwise)"=w476, "OOB in"=w479) -> ("error out"=w473:errorcluster)  [unwired: 7 in, 1 out]
              n140 = Wait (ms)(milliseconds to wait=u32 3000) -> ()  [unwired: 1 out]
            }
          }
          frame Enabled {
          }
        }
        n141 = timed-loop {
          timing: w467 -> [_]
          timing-out: [_] -> w466
          tunnel: w461 -> [w491]
          tunnel: w460 -> [w490]
          tunnel: [w488] -> w454
          tunnel: [w487] -> w453
          tunnel: w446 -> [w486]
          tunnel: [w483] -> w457
          stop <- TRUE stop-if-true
          n142 = for {
            N: 10000 -> [_]
            shift-right: [w503] -> w488
            shift-left: w491 -> [w505]
            shift-right: [w502] -> w487
            shift-left: w490 -> [w504]
            shift-right: [w496] -> w483
            shift-left: 0.0 -> [w497]
            shift-right: [w495] -> _
            shift-left: w486 -> [w501]
            i -> [w493]
            n143 = flat-sequence {
              tunnel: w504 -> [w516]
              tunnel: w505 -> [w517]
              tunnel: [w517] -> w509
              tunnel: [w516] -> w508
              tunnel: [w515] -> w499
              tunnel: w501 -> [w514]
              tunnel: [w514] -> w507
              tunnel: w509 -> [w523]
              tunnel: w508 -> [w521]
              tunnel: [w520] -> w506
              tunnel: w507 -> [w522]
              tunnel: [w519] -> w494
              tunnel: [w518] -> w492
              tunnel: [w540] -> w503
              tunnel: w506 -> [w540]
              tunnel: [w539] -> w502
              tunnel: [w538] -> w500
              tunnel: [w537] -> w495
              tunnel: w494 -> [w537]
              tunnel: w492 -> [w539]
              frame #0 {
                n144 = call <vilib>:"High Resolution Relative Seconds.vi"() -> ("relative seconds"=w515:dbl)
              }
              frame #1 {
                n145 = call "Read OOB DVR.vi"("error in"=w521, "OOB in"=w523) -> ("error out"=w526:errorcluster, "New Commands"=w524:bool, "OOB out"=w525:refnum<class "CIFOutOfBand.lvclass">)  [unwired: 6 in, 1 out]
                n146 = case shown="True" w524 {
                  tunnel: w525 -> [w527 w536]
                  tunnel: w526 -> [w528 w535]
                  tunnel: [w527 w533] -> w520
                  tunnel: w522 -> [_ w531]
                  tunnel: [_ w529] -> w519
                  tunnel: [w528 w530] -> w518
                  frame False {
                  }
                  frame True {
                    n147 = call "Read Local OOB Data.vi"("error in"=w535, "OOB in"=w536) -> ("error out"=w534:errorcluster, "Local OOB Data"=w532:variant, "OOB out"=w533:refnum<class "CIFOutOfBand.lvclass">)  [unwired: 7 in]
                    n148 = Variant To Data(error in=w534, type=w531, Variant=w532) -> (data=w529:T5, error out=w530:errorcluster)
                  }
                }
              }
              frame #2 {
                n149 = call <vilib>:"High Resolution Relative Seconds.vi"() -> ("relative seconds"=w538:dbl)
              }
            }
            n150 = Subtract(x=w500, y=w499) -> (x-y=w498:dbl)
            n151 = case shown="0" w493 {
              tunnel: w498 -> [_ w513]
              tunnel: w497 -> [w510 w512]
              tunnel: [w510 w511] -> w496
              frame 0 {
              }
              frame 1, Default {
                n152 = Max & Min(x=w513, y=w512) -> (max(x,y)=w511:dbl)  [unwired: 1 out]
              }
            }
          }
        }
        "Max no conflict" <- w457
        n153 = node-c288(w468) -> ()  [unwired: 1 out]
        n154 = node-c288(w466) -> ()  [unwired: 1 out]
        n155 = Subtract(x=w465, y=w464) -> (x-y=w463:dbl)
        n156 = Divide(x=w463, y=w462) -> (x/y=w459:dbl)
        "avg no conflict" <- w459
        n157 = Less?(x=w457, y=9e-07) -> (x < y?=w455:bool)
        n158 = Less?(x=w459, y=5e-07) -> ()  [unwired: 1 out]
        n159 = call "Close OOB.vi"("error in"=w453, "OOB in"=w454) -> ("error out"=w452:errorcluster)  [unwired: 9 in]
      }
      frame 4 {
        w600 = u64 0
        n160 = New Data Value Reference(data value=w600, error in=w602) -> (data value reference=w603:refnum<data-value>, error out=w601:errorcluster)
        n161 = node-c288() -> (w618:T1)
        n162 = node-c288() -> (w616:T1)
        n163 = timed-loop {
          timing: w618 -> [_]
          timing-out: [_] -> w617
          tunnel: w603 -> [w686]
          tunnel: w601 -> [w685]
          tunnel: [w681] -> w610
          tunnel: [w679] -> w609
          tunnel: [w677] -> w614
          tunnel: [w676] -> w613
          tunnel: [w675] -> w611
          tunnel: w600 -> [w673]
          stop <- TRUE stop-if-true
          n164 = flat-sequence {
            tunnel: w685 -> [w689]
            tunnel: w686 -> [w690]
            tunnel: [w690] -> w683
            tunnel: [w689] -> w682
            tunnel: [w688] -> w676
            tunnel: w673 -> [w687]
            tunnel: [w687] -> w672
            tunnel: w683 -> [w696]
            tunnel: w682 -> [w695]
            tunnel: [w694] -> w680
            tunnel: [w693] -> w678
            tunnel: [w692] -> w674
            tunnel: w672 -> [w691]
            tunnel: [w705] -> w681
            tunnel: w680 -> [w705]
            tunnel: [w704] -> w679
            tunnel: w678 -> [w704]
            tunnel: [w703] -> w677
            tunnel: [w702] -> w675
            tunnel: w674 -> [w702]
            frame #0 {
              n165 = call <vilib>:"High Resolution Relative Seconds.vi"() -> ("relative seconds"=w688:dbl)
            }
            frame #1 {
              w692 = 10000
              n166 = for {
                N: w692 -> [_]
                shift-right: [w698] -> w694
                shift-left: w696 -> [w700]
                shift-right: [w697] -> w693
                shift-left: w695 -> [_]
                shift-right: [w699] -> _
                shift-left: w691 -> [_]
                n167 = in-place {
                  in-place-border: [w701] -> w699
                  n168 = in-place-dvr #1(w700) -> (w701:u64)  [unwired: 1 out]
                  n169 = in-place-dvr #1(w701) -> (w698:refnum<data-value>, w697:errorcluster)
                }
              }
            }
            frame #2 {
              n170 = call <vilib>:"High Resolution Relative Seconds.vi"() -> ("relative seconds"=w703:dbl)
            }
          }
        }
        n171 = timed-loop {
          timing: w616 -> [_]
          timing-out: [_] -> w615
          tunnel: w610 -> [w632]
          tunnel: w609 -> [w631]
          tunnel: [w629] -> w599
          tunnel: [w628] -> w598
          tunnel: w600 -> [w627]
          tunnel: [w624] -> w606
          stop <- TRUE stop-if-true
          n172 = for {
            N: 10000 -> [_]
            shift-right: [w644] -> w629
            shift-left: w632 -> [w646]
            shift-right: [w643] -> w628
            shift-left: w631 -> [w645]
            shift-right: [w637] -> w624
            shift-left: 0.0 -> [w638]
            shift-right: [w636] -> _
            shift-left: w627 -> [w642]
            i -> [w634]
            n173 = flat-sequence {
              tunnel: w645 -> [w657]
              tunnel: w646 -> [w658]
              tunnel: [w658] -> w650
              tunnel: [w657] -> w649
              tunnel: [w656] -> w640
              tunnel: w642 -> [w655]
              tunnel: [w655] -> w648
              tunnel: w650 -> [w662]
              tunnel: w649 -> [_]
              tunnel: [w660] -> w647
              tunnel: w648 -> [_]
              tunnel: [w661] -> w635
              tunnel: [w659] -> w633
              tunnel: [w667] -> w644
              tunnel: w647 -> [w667]
              tunnel: [w666] -> w643
              tunnel: [w665] -> w641
              tunnel: [w664] -> w636
              tunnel: w635 -> [w664]
              tunnel: w633 -> [w666]
              frame #0 {
                n174 = call <vilib>:"High Resolution Relative Seconds.vi"() -> ("relative seconds"=w656:dbl)
              }
              frame #1 {
                n175 = in-place {
                  in-place-border: [w663] -> w661
                  n176 = in-place-dvr #2(w662) -> (w663:u64)  [unwired: 1 out]
                  n177 = in-place-dvr #2(w663) -> (w660:refnum<data-value>, w659:errorcluster)
                }
              }
              frame #2 {
                n178 = call <vilib>:"High Resolution Relative Seconds.vi"() -> ("relative seconds"=w665:dbl)
              }
            }
            n179 = Subtract(x=w641, y=w640) -> (x-y=w639:dbl)
            n180 = case shown="0" w634 {
              tunnel: w639 -> [_ w654]
              tunnel: w638 -> [w651 w653]
              tunnel: [w651 w652] -> w637
              frame 0 {
              }
              frame 1, Default {
                n181 = Max & Min(x=w654, y=w653) -> (max(x,y)=w652:dbl)  [unwired: 1 out]
              }
            }
          }
        }
        "Max raw dvr" <- w606
        n182 = while {
          tunnel: w603 -> [w622]
          i -> [w621]
          stop <- w619 stop-if-true
          n183 = To Unsigned Quad Integer(1:w621) -> (0:w620:u64)
          n184 = in-place {
            in-place-border: w620 -> [w623]
            n185 = in-place-dvr #3(w622) -> ()  [unwired: 2 out]
            n186 = in-place-dvr #3(w623) -> (w619:errorcluster)  [unwired: 1 out]
          }
        }
        n187 = node-c288(w617) -> ()  [unwired: 1 out]
        n188 = node-c288(w615) -> ()  [unwired: 1 out]
        n189 = Subtract(x=w614, y=w613) -> (x-y=w612:dbl)
        n190 = Divide(x=w612, y=w611) -> (x/y=w608:dbl)
        "avg raw dvr" <- w608
        n191 = Less?(x=w606, y=9e-07) -> (x < y?=w604:bool)
        n192 = Delete Data Value Reference(data value reference=w599, error in=w598) -> (error out=w597:errorcluster)  [unwired: 1 out]
        n193 = Less?(x=w608, y=5e-07) -> ()  [unwired: 1 out]
      }
      frame 5 {
        w713 = u64 0
        n194 = New Data Value Reference(data value=w713, error in=w715) -> (data value reference=w716:refnum<data-value>, error out=w714:errorcluster)
        n195 = node-c288() -> (w731:T1)
        n196 = node-c288() -> (w729:T1)
        n197 = timed-loop {
          timing: w731 -> [_]
          timing-out: [_] -> w730
          tunnel: w716 -> [w804]
          tunnel: w714 -> [w803]
          tunnel: [w799] -> w723
          tunnel: [w797] -> w722
          tunnel: [w795] -> w727
          tunnel: [w794] -> w726
          tunnel: [w793] -> w724
          tunnel: w713 -> [w791]
          stop <- TRUE stop-if-true
          n198 = flat-sequence {
            tunnel: w803 -> [w807]
            tunnel: w804 -> [w808]
            tunnel: [w808] -> w801
            tunnel: [w807] -> w800
            tunnel: [w806] -> w794
            tunnel: w791 -> [w805]
            tunnel: [w805] -> w790
            tunnel: w801 -> [w814]
            tunnel: w800 -> [w813]
            tunnel: [w812] -> w798
            tunnel: [w811] -> w796
            tunnel: [w810] -> w792
            tunnel: w790 -> [w809]
            tunnel: [w825] -> w799
            tunnel: w798 -> [w825]
            tunnel: [w824] -> w797
            tunnel: w796 -> [w824]
            tunnel: [w823] -> w795
            tunnel: [w822] -> w793
            tunnel: w792 -> [w822]
            frame #0 {
              n199 = call <vilib>:"High Resolution Relative Seconds.vi"() -> ("relative seconds"=w806:dbl)
            }
            frame #1 {
              w810 = 10000
              n200 = for {
                N: w810 -> [_]
                shift-right: [w818] -> w812
                shift-left: w814 -> [w820]
                shift-right: [w817] -> w811
                shift-left: w813 -> [_]
                shift-right: [w819] -> _
                shift-left: w809 -> [_]
                i -> [w816]
                n201 = To Unsigned Quad Integer(1:w816) -> (0:w815:u64)
                n202 = in-place {
                  in-place-border: [w821] -> w819
                  in-place-border: w815 -> [w821]
                  n203 = in-place-dvr #4(w820) -> ()  [unwired: 2 out]
                  n204 = in-place-dvr #4(w821) -> (w818:refnum<data-value>, w817:errorcluster)
                }
              }
            }
            frame #2 {
              n205 = call <vilib>:"High Resolution Relative Seconds.vi"() -> ("relative seconds"=w823:dbl)
            }
          }
        }
        n206 = timed-loop {
          timing: w729 -> [_]
          timing-out: [_] -> w728
          tunnel: w723 -> [w746]
          tunnel: w722 -> [w745]
          tunnel: [w743] -> w712
          tunnel: [w742] -> w711
          tunnel: w713 -> [w741]
          tunnel: [w738] -> w719
          stop <- TRUE stop-if-true
          n207 = for {
            N: 10000 -> [_]
            shift-right: [w760] -> w743
            shift-left: w746 -> [w762]
            shift-right: [w759] -> w742
            shift-left: w745 -> [w761]
            shift-right: [w753] -> w738
            shift-left: 0.0 -> [w754]
            shift-right: [w752] -> _
            shift-left: w741 -> [w758]
            i -> [w749]
            n208 = To Unsigned Quad Integer(1:w749) -> (0:w748:u64)
            n209 = flat-sequence {
              tunnel: w761 -> [w774]
              tunnel: w762 -> [w775]
              tunnel: [w775] -> w766
              tunnel: [w774] -> w765
              tunnel: [w773] -> w756
              tunnel: w758 -> [w772]
              tunnel: [w772] -> w764
              tunnel: w748 -> [w771]
              tunnel: [w771] -> w747
              tunnel: w766 -> [w780]
              tunnel: w765 -> [_]
              tunnel: [w778] -> w763
              tunnel: w764 -> [_]
              tunnel: [w779] -> w751
              tunnel: [w777] -> w750
              tunnel: w747 -> [w776]
              tunnel: [w785] -> w760
              tunnel: w763 -> [w785]
              tunnel: [w784] -> w759
              tunnel: [w783] -> w757
              tunnel: [w782] -> w752
              tunnel: w751 -> [w782]
              tunnel: w750 -> [w784]
              frame #0 {
                n210 = call <vilib>:"High Resolution Relative Seconds.vi"() -> ("relative seconds"=w773:dbl)
              }
              frame #1 {
                n211 = in-place {
                  in-place-border: [w781] -> w779
                  in-place-border: w776 -> [w781]
                  n212 = in-place-dvr #5(w780) -> ()  [unwired: 2 out]
                  n213 = in-place-dvr #5(w781) -> (w778:refnum<data-value>, w777:errorcluster)
                }
              }
              frame #2 {
                n214 = call <vilib>:"High Resolution Relative Seconds.vi"() -> ("relative seconds"=w783:dbl)
              }
            }
            n215 = Subtract(x=w757, y=w756) -> (x-y=w755:dbl)
            n216 = case shown="0" w749 {
              tunnel: w755 -> [_ w770]
              tunnel: w754 -> [w767 w769]
              tunnel: [w767 w768] -> w753
              frame 0 {
              }
              frame 1, Default {
                n217 = Max & Min(x=w770, y=w769) -> (max(x,y)=w768:dbl)  [unwired: 1 out]
              }
            }
          }
        }
        "Max raw dvr write" <- w719
        n218 = while {
          tunnel: w716 -> [w736]
          tunnel: [w732] -> _
          i -> [w735]
          stop <- w733 stop-if-true
          n219 = To Unsigned Quad Integer(1:w735) -> (0:w734:u64)
          n220 = in-place {
            in-place-border: w734 -> [_]
            in-place-border: [w737] -> w732
            n221 = in-place-dvr #6(w736) -> (w737:u64)  [unwired: 1 out]
            n222 = in-place-dvr #6(w737) -> (w733:errorcluster)  [unwired: 1 out]
          }
        }
        n223 = node-c288(w730) -> ()  [unwired: 1 out]
        n224 = node-c288(w728) -> ()  [unwired: 1 out]
        n225 = Subtract(x=w727, y=w726) -> (x-y=w725:dbl)
        n226 = Divide(x=w725, y=w724) -> (x/y=w721:dbl)
        "avg raw dvr write" <- w721
        n227 = Less?(x=w719, y=9e-07) -> (x < y?=w717:bool)
        n228 = Delete Data Value Reference(data value reference=w712, error in=w711) -> (error out=w710:errorcluster)  [unwired: 1 out]
        n229 = Less?(x=w721, y=5e-07) -> ()  [unwired: 1 out]
      }
      frame 6 {
        w834 = u64 0
        n230 = RT FIFO Create(1:w834, 3:w832, 7:T4 {"read mode"=enum."polling", "write mode"=enum."blocking"} ("r/w modes (polling,polling)")) -> (8:w833:refnum<k33>, 11:w831:errorcluster)  [unwired: 5 in, 1 out]
        n231 = node-c288() -> (w852:T1)
        n232 = node-c288() -> (w850:T1)
        n233 = timed-loop {
          timing: w852 -> [_]
          timing-out: [_] -> w851
          tunnel: w833 -> [w923]
          tunnel: w831 -> [w922]
          tunnel: [w918] -> w844
          tunnel: [w916] -> w843
          tunnel: [w914] -> w848
          tunnel: [w913] -> w847
          tunnel: [w912] -> w845
          tunnel: w834 -> [w910]
          stop <- TRUE stop-if-true
          n234 = flat-sequence {
            tunnel: w922 -> [w926]
            tunnel: w923 -> [w927]
            tunnel: [w927] -> w920
            tunnel: [w926] -> w919
            tunnel: [w925] -> w913
            tunnel: w910 -> [w924]
            tunnel: [w924] -> w909
            tunnel: w920 -> [w933]
            tunnel: w919 -> [w932]
            tunnel: [w931] -> w917
            tunnel: [w930] -> w915
            tunnel: [w929] -> w911
            tunnel: w909 -> [w928]
            tunnel: [w944] -> w918
            tunnel: w917 -> [w944]
            tunnel: [w943] -> w916
            tunnel: w915 -> [w943]
            tunnel: [w942] -> w914
            tunnel: [w941] -> w912
            tunnel: w911 -> [w941]
            frame #0 {
              n235 = call <vilib>:"High Resolution Relative Seconds.vi"() -> ("relative seconds"=w925:dbl)
            }
            frame #1 {
              w929 = 10000
              n236 = for {
                N: w929 -> [_]
                shift-right: [w938] -> w931
                shift-left: w933 -> [w939]
                shift-right: [w934] -> w930
                shift-left: w932 -> [w937]
                shift-right: [w935] -> _
                shift-left: w928 -> [w936]
                i -> [w940]
                n237 = To Unsigned Quad Integer(1:w940) -> ()  [unwired: 1 out]
                n238 = RT FIFO Read(0:w939, 1:w936, 3:w937) -> (8:w938:refnum<k33>, 9:w935:u64, 11:w934:errorcluster)  [unwired: 1 in, 2 out]
              }
            }
            frame #2 {
              n239 = call <vilib>:"High Resolution Relative Seconds.vi"() -> ("relative seconds"=w942:dbl)
            }
          }
        }
        n240 = timed-loop {
          timing: w850 -> [_]
          timing-out: [_] -> w849
          tunnel: w844 -> [w865]
          tunnel: w843 -> [w864]
          tunnel: [w862] -> w837
          tunnel: [w861] -> w836
          tunnel: w834 -> [w860]
          tunnel: [w857] -> w840
          stop <- TRUE stop-if-true
          n241 = for {
            N: 10000 -> [_]
            shift-right: [w879] -> w862
            shift-left: w865 -> [w881]
            shift-right: [w878] -> w861
            shift-left: w864 -> [w880]
            shift-right: [w872] -> w857
            shift-left: 0.0 -> [w873]
            shift-right: [w871] -> _
            shift-left: w860 -> [w877]
            i -> [w868]
            n242 = To Unsigned Quad Integer(1:w868) -> (0:w867:u64)
            n243 = flat-sequence {
              tunnel: w880 -> [w893]
              tunnel: w881 -> [w894]
              tunnel: [w894] -> w885
              tunnel: [w893] -> w884
              tunnel: [w892] -> w875
              tunnel: w877 -> [w891]
              tunnel: [w891] -> w883
              tunnel: w867 -> [w890]
              tunnel: [w890] -> w866
              tunnel: w885 -> [w900]
              tunnel: w884 -> [w898]
              tunnel: [w899] -> w882
              tunnel: w883 -> [w897]
              tunnel: [w896] -> w870
              tunnel: [w895] -> w869
              tunnel: w866 -> [_]
              tunnel: [w904] -> w879
              tunnel: w882 -> [w904]
              tunnel: [w903] -> w878
              tunnel: [w902] -> w876
              tunnel: [w901] -> w871
              tunnel: w870 -> [w901]
              tunnel: w869 -> [w903]
              frame #0 {
                n244 = call <vilib>:"High Resolution Relative Seconds.vi"() -> ("relative seconds"=w892:dbl)
              }
              frame #1 {
                n245 = RT FIFO Read(0:w900, 1:w897, 3:w898) -> (8:w899:refnum<k33>, 9:w896:u64, 11:w895:errorcluster)  [unwired: 1 in, 2 out]
              }
              frame #2 {
                n246 = call <vilib>:"High Resolution Relative Seconds.vi"() -> ("relative seconds"=w902:dbl)
              }
            }
            n247 = Subtract(x=w876, y=w875) -> (x-y=w874:dbl)
            n248 = case shown="0" w868 {
              tunnel: w874 -> [_ w889]
              tunnel: w873 -> [w886 w888]
              tunnel: [w886 w887] -> w872
              frame 0 {
              }
              frame 1, Default {
                n249 = Max & Min(x=w889, y=w888) -> (max(x,y)=w887:dbl)  [unwired: 1 out]
              }
            }
          }
        }
        "Max RTFifo" <- w840
        n250 = while {
          tunnel: w833 -> [w855]
          i -> [w856]
          stop <- w853 stop-if-true
          n251 = To Unsigned Quad Integer(1:w856) -> (0:w854:u64)
          n252 = RT FIFO Write(0:w855, 1:w854) -> (11:w853:errorcluster)  [unwired: 3 in, 3 out]
        }
        n253 = node-c288(w851) -> ()  [unwired: 1 out]
        n254 = node-c288(w849) -> ()  [unwired: 1 out]
        n255 = Subtract(x=w848, y=w847) -> (x-y=w846:dbl)
        n256 = Divide(x=w846, y=w845) -> (x/y=w842:dbl)
        "avg RTFifo" <- w842
        n257 = Less?(x=w840, y=9e-07) -> (x < y?=w838:bool)
        n258 = RT FIFO Delete(0:w837, 3:w836) -> (11:w835:errorcluster)  [unwired: 1 in]
        n259 = Less?(x=w842, y=5e-07) -> ()  [unwired: 1 out]
      }
      frame 7 {
        w952 = u64 0
        n260 = Obtain Notifier(notification data type=w952, error in (no error)=w950) -> (notifier out=w951:refnum<notifier>, error out=w949:errorcluster)  [unwired: 2 in, 1 out]
        n261 = node-c288() -> (w970:T1)
        n262 = node-c288() -> (w968:T1)
        n263 = timed-loop {
          timing: w970 -> [_]
          timing-out: [_] -> w969
          tunnel: w951 -> [w1041]
          tunnel: w949 -> [w1040]
          tunnel: [w1036] -> w962
          tunnel: [w1034] -> w961
          tunnel: [w1032] -> w966
          tunnel: [w1031] -> w965
          tunnel: [w1030] -> w963
          tunnel: w952 -> [w1028]
          stop <- TRUE stop-if-true
          n264 = flat-sequence {
            tunnel: w1040 -> [w1044]
            tunnel: w1041 -> [w1045]
            tunnel: [w1045] -> w1038
            tunnel: [w1044] -> w1037
            tunnel: [w1043] -> w1031
            tunnel: w1028 -> [w1042]
            tunnel: [w1042] -> w1027
            tunnel: w1038 -> [w1051]
            tunnel: w1037 -> [w1050]
            tunnel: [w1049] -> w1035
            tunnel: [w1048] -> w1033
            tunnel: [w1047] -> w1029
            tunnel: w1027 -> [w1046]
            tunnel: [w1062] -> w1036
            tunnel: w1035 -> [w1062]
            tunnel: [w1061] -> w1034
            tunnel: w1033 -> [w1061]
            tunnel: [w1060] -> w1032
            tunnel: [w1059] -> w1030
            tunnel: w1029 -> [w1059]
            frame #0 {
              n265 = call <vilib>:"High Resolution Relative Seconds.vi"() -> ("relative seconds"=w1043:dbl)
            }
            frame #1 {
              w1047 = 10000
              n266 = for {
                N: w1047 -> [_]
                shift-right: [w1056] -> w1049
                shift-left: w1051 -> [w1057]
                shift-right: [w1053] -> w1048
                shift-left: w1050 -> [w1055]
                shift-right: [w1054] -> _
                shift-left: w1046 -> [_]
                i -> [w1058]
                n267 = To Unsigned Quad Integer(1:w1058) -> ()  [unwired: 1 out]
                n268 = Wait on Notification(notifier=w1057, timeout in ms (-1)=0, error in (no error)=w1055) -> (notifier out=w1056:refnum<notifier>, notification=w1054:u64, error out=w1053:errorcluster)  [unwired: 1 in, 1 out]
              }
            }
            frame #2 {
              n269 = call <vilib>:"High Resolution Relative Seconds.vi"() -> ("relative seconds"=w1060:dbl)
            }
          }
        }
        n270 = timed-loop {
          timing: w968 -> [_]
          timing-out: [_] -> w967
          tunnel: w962 -> [w983]
          tunnel: w961 -> [w982]
          tunnel: [w980] -> w955
          tunnel: [w979] -> w954
          tunnel: w952 -> [w978]
          tunnel: [w975] -> w958
          stop <- TRUE stop-if-true
          n271 = for {
            N: 10000 -> [_]
            shift-right: [w997] -> w980
            shift-left: w983 -> [w999]
            shift-right: [w996] -> w979
            shift-left: w982 -> [w998]
            shift-right: [w990] -> w975
            shift-left: 0.0 -> [w991]
            shift-right: [w989] -> _
            shift-left: w978 -> [w995]
            i -> [w986]
            n272 = To Unsigned Quad Integer(1:w986) -> (0:w985:u64)
            n273 = flat-sequence {
              tunnel: w998 -> [w1011]
              tunnel: w999 -> [w1012]
              tunnel: [w1012] -> w1003
              tunnel: [w1011] -> w1002
              tunnel: [w1010] -> w993
              tunnel: w995 -> [w1009]
              tunnel: [w1009] -> w1001
              tunnel: w985 -> [w1008]
              tunnel: [w1008] -> w984
              tunnel: w1003 -> [w1018]
              tunnel: w1002 -> [w1016]
              tunnel: [w1017] -> w1000
              tunnel: w1001 -> [_]
              tunnel: [w1015] -> w988
              tunnel: [w1014] -> w987
              tunnel: w984 -> [_]
              tunnel: [w1022] -> w997
              tunnel: w1000 -> [w1022]
              tunnel: [w1021] -> w996
              tunnel: [w1020] -> w994
              tunnel: [w1019] -> w989
              tunnel: w988 -> [w1019]
              tunnel: w987 -> [w1021]
              frame #0 {
                n274 = call <vilib>:"High Resolution Relative Seconds.vi"() -> ("relative seconds"=w1010:dbl)
              }
              frame #1 {
                n275 = Wait on Notification(notifier=w1018, timeout in ms (-1)=0, error in (no error)=w1016) -> (notifier out=w1017:refnum<notifier>, notification=w1015:u64, error out=w1014:errorcluster)  [unwired: 1 in, 1 out]
              }
              frame #2 {
                n276 = call <vilib>:"High Resolution Relative Seconds.vi"() -> ("relative seconds"=w1020:dbl)
              }
            }
            n277 = Subtract(x=w994, y=w993) -> (x-y=w992:dbl)
            n278 = case shown="0" w986 {
              tunnel: w992 -> [_ w1007]
              tunnel: w991 -> [w1004 w1006]
              tunnel: [w1004 w1005] -> w990
              frame 0 {
              }
              frame 1, Default {
                n279 = Max & Min(x=w1007, y=w1006) -> (max(x,y)=w1005:dbl)  [unwired: 1 out]
              }
            }
          }
        }
        "Max Notifier" <- w958
        n280 = while {
          tunnel: w951 -> [w973]
          i -> [w974]
          stop <- w971 stop-if-true
          n281 = To Unsigned Quad Integer(1:w974) -> (0:w972:u64)
          n282 = Send Notification(notification=w972, notifier=w973) -> (error out=w971:errorcluster)  [unwired: 1 in, 1 out]
        }
        n283 = node-c288(w969) -> ()  [unwired: 1 out]
        n284 = node-c288(w967) -> ()  [unwired: 1 out]
        n285 = Subtract(x=w966, y=w965) -> (x-y=w964:dbl)
        n286 = Divide(x=w964, y=w963) -> (x/y=w960:dbl)
        "avg Notifier" <- w960
        n287 = Less?(x=w958, y=9e-07) -> (x < y?=w956:bool)
        n288 = Release Notifier(notifier=w955, error in (no error)=w954) -> (error out=w953:errorcluster)  [unwired: 1 in, 2 out]
        n289 = Less?(x=w960, y=5e-07) -> ()  [unwired: 1 out]
      }
      frame 8 {
        w1072 = u64 0
        n290 = Generate Occurrence() -> (w1071:refnum<k4>)
        n291 = flat-sequence {
          tunnel: [w1091] -> w1068
          frame #0 {
            w1091 = FALSE ("stop")
            n292 = local write "stop"(w1091) -> ()
          }
        }
        n293 = node-c288() -> (w1087:T1)
        n294 = node-c288() -> (w1085:T1)
        n295 = timed-loop {
          timing: w1087 -> [_]
          timing-out: [_] -> w1086
          tunnel: w1071 -> [w1157]
          tunnel: w1070 -> [w1156]
          tunnel: [w1152] -> w1079
          tunnel: [w1150] -> w1078
          tunnel: [w1148] -> w1083
          tunnel: [w1147] -> w1082
          tunnel: [w1146] -> w1080
          tunnel: w1072 -> [w1144]
          stop <- TRUE stop-if-true
          n296 = flat-sequence {
            tunnel: w1156 -> [w1160]
            tunnel: w1157 -> [w1161]
            tunnel: [w1161] -> w1154
            tunnel: [w1160] -> w1153
            tunnel: [w1159] -> w1147
            tunnel: w1144 -> [w1158]
            tunnel: [w1158] -> w1143
            tunnel: w1154 -> [w1167]
            tunnel: w1153 -> [w1166]
            tunnel: [w1165] -> w1151
            tunnel: [w1164] -> w1149
            tunnel: [w1163] -> w1145
            tunnel: w1143 -> [w1162]
            tunnel: [w1176] -> w1152
            tunnel: w1151 -> [w1176]
            tunnel: [w1175] -> w1150
            tunnel: w1149 -> [w1175]
            tunnel: [w1174] -> w1148
            tunnel: [w1173] -> w1146
            tunnel: w1145 -> [w1173]
            frame #0 {
              n297 = call <vilib>:"High Resolution Relative Seconds.vi"() -> ("relative seconds"=w1159:dbl)
            }
            frame #1 {
              w1163 = 10000
              n298 = for {
                N: w1163 -> [_]
                shift-right: [w1169] -> w1165
                shift-left: w1167 -> [w1169]
                shift-right: [w1170] -> w1164
                shift-left: w1166 -> [w1170]
                shift-right: [w1168] -> _
                shift-left: w1162 -> [w1168]
                i -> [w1172]
                n299 = To Unsigned Quad Integer(1:w1172) -> ()  [unwired: 1 out]
                n300 = Wait on Occurrence(2:w1169, 3:0 ("timeout in ms (-1)")) -> ()  [unwired: 1 in, 1 out]
              }
            }
            frame #2 {
              n301 = call <vilib>:"High Resolution Relative Seconds.vi"() -> ("relative seconds"=w1174:dbl)
            }
          }
        }
        n302 = timed-loop {
          timing: w1085 -> [_]
          timing-out: [_] -> w1084
          tunnel: w1079 -> [w1101]
          tunnel: w1078 -> [w1100]
          tunnel: [w1098] -> _
          tunnel: [w1097] -> w1069
          tunnel: w1072 -> [w1096]
          tunnel: [w1093] -> w1075
          tunnel: [TRUE] -> w1067
          stop <- TRUE stop-if-true
          n303 = for {
            N: 10000 -> [_]
            shift-right: [w1115] -> w1098
            shift-left: w1101 -> [w1117]
            shift-right: [w1114] -> w1097
            shift-left: w1100 -> [w1116]
            shift-right: [w1108] -> w1093
            shift-left: 0.0 -> [w1109]
            shift-right: [w1107] -> _
            shift-left: w1096 -> [w1113]
            i -> [w1104]
            n304 = To Unsigned Quad Integer(1:w1104) -> (0:w1103:u64)
            n305 = flat-sequence {
              tunnel: w1116 -> [w1129]
              tunnel: w1117 -> [w1130]
              tunnel: [w1130] -> w1121
              tunnel: [w1129] -> w1120
              tunnel: [w1128] -> w1111
              tunnel: w1113 -> [w1127]
              tunnel: [w1127] -> w1119
              tunnel: w1103 -> [w1126]
              tunnel: [w1126] -> w1102
              tunnel: w1121 -> [w1134]
              tunnel: w1120 -> [w1132]
              tunnel: [w1134] -> w1118
              tunnel: w1119 -> [w1131]
              tunnel: [w1131] -> w1106
              tunnel: [w1132] -> w1105
              tunnel: w1102 -> [_]
              tunnel: [w1138] -> w1115
              tunnel: w1118 -> [w1138]
              tunnel: [w1137] -> w1114
              tunnel: [w1136] -> w1112
              tunnel: [w1135] -> w1107
              tunnel: w1106 -> [w1135]
              tunnel: w1105 -> [w1137]
              frame #0 {
                n306 = call <vilib>:"High Resolution Relative Seconds.vi"() -> ("relative seconds"=w1128:dbl)
              }
              frame #1 {
                n307 = Wait on Occurrence(2:w1134, 3:0 ("timeout in ms (-1)")) -> ()  [unwired: 1 in, 1 out]
              }
              frame #2 {
                n308 = call <vilib>:"High Resolution Relative Seconds.vi"() -> ("relative seconds"=w1136:dbl)
              }
            }
            n309 = Subtract(x=w1112, y=w1111) -> (x-y=w1110:dbl)
            n310 = case shown="0" w1104 {
              tunnel: w1110 -> [_ w1125]
              tunnel: w1109 -> [w1122 w1124]
              tunnel: [w1122 w1123] -> w1108
              frame 0 {
              }
              frame 1, Default {
                n311 = Max & Min(x=w1125, y=w1124) -> (max(x,y)=w1123:dbl)  [unwired: 1 out]
              }
            }
          }
        }
        "Max Occur" <- w1075
        n312 = while {
          tunnel: w1071 -> [w1089]
          tunnel: w1068 -> [_]
          i -> [w1090]
          stop <- w1088 stop-if-true
          n313 = To Unsigned Quad Integer(1:w1090) -> ()  [unwired: 1 out]
          n314 = Set Occurrence(w1089) -> ()
          n315 = local read "stop"() -> (w1088:bool)
        }
        n316 = node-c288(w1086) -> ()  [unwired: 1 out]
        n317 = node-c288(w1084) -> ()  [unwired: 1 out]
        n318 = local write "stop"(w1067) -> ()
        n319 = Subtract(x=w1083, y=w1082) -> (x-y=w1081:dbl)
        n320 = Divide(x=w1081, y=w1080) -> (x/y=w1077:dbl)
        "avg Occur" <- w1077
        n321 = Less?(x=w1075, y=9e-07) -> (x < y?=w1073:bool)
        n322 = Less?(x=w1077, y=5e-07) -> ()  [unwired: 1 out]
      }
      frame 9 {
        w1187 = T5 {"Numeric"=54.0, "Array"=[{"Numeric"=3.1415, "String"="strings are fun especially when they are pretty long. a;lfkjasd;lkfjsd;lkfjsd;lkfj;dslkfj ;dslkjf f;ldskjff ;dskfj;s dlkfj;dslk jfj;dslkk jfs\ndsajf'sdjkf ;dsaf\nsjd f'\nsdafkjj'lds kf sda\nf jdsa'", "Boolean"=FALSE}, {"Numeric"=-6554654654564.0, "String"="safdsfa", "Boolean"=FALSE}, {"Numeric"=1e+20, "String"="asdfasd", "Boolean"=FALSE}, {"Numeric"=2.0, "String"="afd", "Boolean"=TRUE}, {"Numeric"=12.34, "String"="data", "Boolean"=FALSE}], "string"="strings", "Null array"=[0]} ("Test Config")
        n323 = Obtain Notifier(notification data type=w1187, error in (no error)=w1186) -> (notifier out=w1184:refnum<notifier>, error out=w1185:errorcluster)  [unwired: 2 in, 1 out]
        n324 = node-c288() -> (w1202:T1)
        n325 = node-c288() -> (w1200:T1)
        n326 = timed-loop {
          timing: w1202 -> [_]
          timing-out: [_] -> w1201
          tunnel: w1184 -> [w1271]
          tunnel: w1185 -> [w1270]
          tunnel: [w1266] -> w1194
          tunnel: [w1264] -> w1193
          tunnel: [w1262] -> w1198
          tunnel: [w1261] -> w1197
          tunnel: [w1260] -> w1195
          tunnel: w1187 -> [w1258]
          stop <- TRUE stop-if-true
          n327 = flat-sequence {
            tunnel: w1270 -> [w1274]
            tunnel: w1271 -> [w1275]
            tunnel: [w1275] -> w1268
            tunnel: [w1274] -> w1267
            tunnel: [w1273] -> w1261
            tunnel: w1258 -> [w1272]
            tunnel: [w1272] -> w1257
            tunnel: w1268 -> [w1281]
            tunnel: w1267 -> [w1280]
            tunnel: [w1279] -> w1265
            tunnel: [w1278] -> w1263
            tunnel: [w1277] -> w1259
            tunnel: w1257 -> [w1276]
            tunnel: [w1291] -> w1266
            tunnel: w1265 -> [w1291]
            tunnel: [w1290] -> w1264
            tunnel: w1263 -> [w1290]
            tunnel: [w1289] -> w1262
            tunnel: [w1288] -> w1260
            tunnel: w1259 -> [w1288]
            frame #0 {
              n328 = call <vilib>:"High Resolution Relative Seconds.vi"() -> ("relative seconds"=w1273:dbl)
            }
            frame #1 {
              w1277 = 10000
              n329 = for {
                N: w1277 -> [_]
                shift-right: [w1286] -> w1279
                shift-left: w1281 -> [w1287]
                shift-right: [w1285] -> w1278
                shift-left: w1280 -> [w1284]
                shift-right: [w1283] -> _
                shift-left: w1276 -> [_]
                n330 = Wait on Notification(notifier=w1287, timeout in ms (-1)=0, error in (no error)=w1284) -> (notifier out=w1286:refnum<notifier>, notification=w1283:T5, error out=w1285:errorcluster)  [unwired: 1 in, 1 out]
              }
            }
            frame #2 {
              n331 = call <vilib>:"High Resolution Relative Seconds.vi"() -> ("relative seconds"=w1289:dbl)
            }
          }
        }
        n332 = timed-loop {
          timing: w1200 -> [_]
          timing-out: [_] -> w1199
          tunnel: w1194 -> [w1216]
          tunnel: w1193 -> [w1215]
          tunnel: [w1213] -> w1183
          tunnel: [w1212] -> w1182
          tunnel: w1187 -> [w1211]
          tunnel: [w1208] -> w1190
          stop <- TRUE stop-if-true
          n333 = for {
            N: 10000 -> [_]
            shift-right: [w1228] -> w1213
            shift-left: w1216 -> [w1230]
            shift-right: [w1227] -> w1212
            shift-left: w1215 -> [w1229]
            shift-right: [w1221] -> w1208
            shift-left: 0.0 -> [w1222]
            shift-right: [w1220] -> _
            shift-left: w1211 -> [w1226]
            i -> [w1218]
            n334 = flat-sequence {
              tunnel: w1229 -> [w1241]
              tunnel: w1230 -> [w1242]
              tunnel: [w1242] -> w1234
              tunnel: [w1241] -> w1233
              tunnel: [w1240] -> w1224
              tunnel: w1226 -> [w1239]
              tunnel: [w1239] -> w1232
              tunnel: w1234 -> [w1248]
              tunnel: w1233 -> [w1245]
              tunnel: [w1247] -> w1231
              tunnel: w1232 -> [_]
              tunnel: [w1244] -> w1219
              tunnel: [w1246] -> w1217
              tunnel: [w1252] -> w1228
              tunnel: w1231 -> [w1252]
              tunnel: [w1251] -> w1227
              tunnel: [w1250] -> w1225
              tunnel: [w1249] -> w1220
              tunnel: w1219 -> [w1249]
              tunnel: w1217 -> [w1251]
              frame #0 {
                n335 = call <vilib>:"High Resolution Relative Seconds.vi"() -> ("relative seconds"=w1240:dbl)
              }
              frame #1 {
                n336 = Wait on Notification(notifier=w1248, timeout in ms (-1)=0, error in (no error)=w1245) -> (notifier out=w1247:refnum<notifier>, notification=w1244:T5, error out=w1246:errorcluster)  [unwired: 1 in, 1 out]
              }
              frame #2 {
                n337 = call <vilib>:"High Resolution Relative Seconds.vi"() -> ("relative seconds"=w1250:dbl)
              }
            }
            n338 = Subtract(x=w1225, y=w1224) -> (x-y=w1223:dbl)
            n339 = case shown="0" w1218 {
              tunnel: w1223 -> [_ w1238]
              tunnel: w1222 -> [w1235 w1237]
              tunnel: [w1235 w1236] -> w1221
              frame 0 {
              }
              frame 1, Default {
                n340 = Max & Min(x=w1238, y=w1237) -> (max(x,y)=w1236:dbl)  [unwired: 1 out]
              }
            }
          }
        }
        "Max Complexnote" <- w1190
        n341 = while {
          tunnel: w1184 -> [w1205]
          tunnel: w1187 -> [w1206]
          i -> [w1207]
          stop <- w1203 stop-if-true
          n342 = Bundle By Name(cluster=w1206, "Numeric"=w1207) -> (w1204:T5)
          n343 = Send Notification(notification=w1204, notifier=w1205) -> (error out=w1203:errorcluster)  [unwired: 1 in, 1 out]
        }
        n344 = node-c288(w1201) -> ()  [unwired: 1 out]
        n345 = node-c288(w1199) -> ()  [unwired: 1 out]
        n346 = Subtract(x=w1198, y=w1197) -> (x-y=w1196:dbl)
        n347 = Divide(x=w1196, y=w1195) -> (x/y=w1192:dbl)
        "avg complexnote" <- w1192
        n348 = Less?(x=w1190, y=4e-05) -> (x < y?=w1188:bool)
        n349 = Less?(x=w1192, y=5e-07) -> ()  [unwired: 1 out]
        n350 = Release Notifier(notifier=w1183, error in (no error)=w1182) -> (error out=w1181:errorcluster)  [unwired: 1 in, 2 out]
      }
      frame 10 {
        w1302 = T5 {"Numeric"=54.0, "Array"=[{"Numeric"=3.1415, "String"="strings are fun especially when they are pretty long. a;lfkjasd;lkfjsd;lkfjsd;lkfj;dslkfj ;dslkjf f;ldskjff ;dskfj;s dlkfj;dslk jfj;dslkk jfs\ndsajf'sdjkf ;dsaf\nsjd f'\nsdafkjj'lds kf sda\nf jdsa'", "Boolean"=FALSE}, {"Numeric"=-6554654654564.0, "String"="safdsfa", "Boolean"=FALSE}, {"Numeric"=1e+20, "String"="asdfasd", "Boolean"=FALSE}, {"Numeric"=2.0, "String"="afd", "Boolean"=TRUE}, {"Numeric"=12.34, "String"="data", "Boolean"=FALSE}], "string"="strings", "Null array"=[0]} ("Test Config")
        n351 = Obtain Notifier(notification data type=w1302, error in (no error)=w1301) -> (notifier out=w1299:refnum<notifier>, error out=w1300:errorcluster)  [unwired: 2 in, 1 out]
        n352 = node-c288() -> (w1317:T1)
        n353 = node-c288() -> (w1315:T1)
        n354 = timed-loop {
          timing: w1317 -> [_]
          timing-out: [_] -> w1316
          tunnel: w1299 -> [w1386]
          tunnel: w1300 -> [w1385]
          tunnel: [w1381] -> w1309
          tunnel: [w1379] -> w1308
          tunnel: [w1377] -> w1313
          tunnel: [w1376] -> w1312
          tunnel: [w1375] -> w1310
          tunnel: w1302 -> [w1373]
          stop <- TRUE stop-if-true
          n355 = flat-sequence {
            tunnel: w1385 -> [w1389]
            tunnel: w1386 -> [w1390]
            tunnel: [w1390] -> w1383
            tunnel: [w1389] -> w1382
            tunnel: [w1388] -> w1376
            tunnel: w1373 -> [w1387]
            tunnel: [w1387] -> w1372
            tunnel: w1383 -> [w1396]
            tunnel: w1382 -> [w1395]
            tunnel: [w1394] -> w1380
            tunnel: [w1393] -> w1378
            tunnel: [w1392] -> w1374
            tunnel: w1372 -> [w1391]
            tunnel: [w1405] -> w1381
            tunnel: w1380 -> [w1405]
            tunnel: [w1404] -> w1379
            tunnel: w1378 -> [w1404]
            tunnel: [w1403] -> w1377
            tunnel: [w1402] -> w1375
            tunnel: w1374 -> [w1402]
            frame #0 {
              n356 = call <vilib>:"High Resolution Relative Seconds.vi"() -> ("relative seconds"=w1388:dbl)
            }
            frame #1 {
              w1392 = 10000
              n357 = for {
                N: w1392 -> [_]
                shift-right: [w1398] -> w1394
                shift-left: w1396 -> [w1401]
                shift-right: [w1399] -> w1393
                shift-left: w1395 -> [w1400]
                shift-right: [w1397] -> _
                shift-left: w1391 -> [w1397]
                n358 = Send Notification(notification=w1397, notifier=w1401, error in (no error)=w1400) -> (notifier out=w1398:refnum<notifier>, error out=w1399:errorcluster)
              }
            }
            frame #2 {
              n359 = call <vilib>:"High Resolution Relative Seconds.vi"() -> ("relative seconds"=w1403:dbl)
            }
          }
        }
        n360 = timed-loop {
          timing: w1315 -> [_]
          timing-out: [_] -> w1314
          tunnel: w1309 -> [w1332]
          tunnel: w1308 -> [w1331]
          tunnel: [w1329] -> w1298
          tunnel: [w1328] -> w1297
          tunnel: w1302 -> [w1327]
          tunnel: [w1324] -> w1305
          stop <- TRUE stop-if-true
          n361 = for {
            N: 10000 -> [_]
            shift-right: [w1344] -> w1329
            shift-left: w1332 -> [w1346]
            shift-right: [w1343] -> w1328
            shift-left: w1331 -> [w1345]
            shift-right: [w1337] -> w1324
            shift-left: 0.0 -> [w1338]
            shift-right: [w1336] -> _
            shift-left: w1327 -> [w1342]
            i -> [w1334]
            n362 = flat-sequence {
              tunnel: w1345 -> [w1357]
              tunnel: w1346 -> [w1358]
              tunnel: [w1358] -> w1350
              tunnel: [w1357] -> w1349
              tunnel: [w1356] -> w1340
              tunnel: w1342 -> [w1355]
              tunnel: [w1355] -> w1348
              tunnel: w1350 -> [w1363]
              tunnel: w1349 -> [w1362]
              tunnel: [w1360] -> w1347
              tunnel: w1348 -> [w1359]
              tunnel: [w1359] -> w1335
              tunnel: [w1361] -> w1333
              tunnel: [w1367] -> w1344
              tunnel: w1347 -> [w1367]
              tunnel: [w1366] -> w1343
              tunnel: [w1365] -> w1341
              tunnel: [w1364] -> w1336
              tunnel: w1335 -> [w1364]
              tunnel: w1333 -> [w1366]
              frame #0 {
                n363 = call <vilib>:"High Resolution Relative Seconds.vi"() -> ("relative seconds"=w1356:dbl)
              }
              frame #1 {
                n364 = Send Notification(notification=w1359, notifier=w1363, error in (no error)=w1362) -> (notifier out=w1360:refnum<notifier>, error out=w1361:errorcluster)
              }
              frame #2 {
                n365 = call <vilib>:"High Resolution Relative Seconds.vi"() -> ("relative seconds"=w1365:dbl)
              }
            }
            n366 = Subtract(x=w1341, y=w1340) -> (x-y=w1339:dbl)
            n367 = case shown="0" w1334 {
              tunnel: w1339 -> [_ w1354]
              tunnel: w1338 -> [w1351 w1353]
              tunnel: [w1351 w1352] -> w1337
              frame 0 {
              }
              frame 1, Default {
                n368 = Max & Min(x=w1354, y=w1353) -> (max(x,y)=w1352:dbl)  [unwired: 1 out]
              }
            }
          }
        }
        "Max Complexnote write" <- w1305
        n369 = while {
          tunnel: w1299 -> [w1321]
          tunnel: w1302 -> [w1322]
          tunnel: [w1319] -> _
          i -> [w1323]
          stop <- w1320 stop-if-true
          n370 = Bundle By Name(cluster=w1322, "Numeric"=w1323) -> ()  [unwired: 1 out]
          n371 = Wait on Notification(notifier=w1321, timeout in ms (-1)=0) -> (notification=w1319:T5, error out=w1320:errorcluster)  [unwired: 2 in, 2 out]
        }
        n372 = node-c288(w1316) -> ()  [unwired: 1 out]
        n373 = node-c288(w1314) -> ()  [unwired: 1 out]
        n374 = Subtract(x=w1313, y=w1312) -> (x-y=w1311:dbl)
        n375 = Divide(x=w1311, y=w1310) -> (x/y=w1307:dbl)
        "avg complexnote write" <- w1307
        n376 = Less?(x=w1305, y=4e-05) -> (x < y?=w1303:bool)
        n377 = Less?(x=w1307, y=5e-07) -> ()  [unwired: 1 out]
        n378 = Release Notifier(notifier=w1298, error in (no error)=w1297) -> (error out=w1296:errorcluster)  [unwired: 1 in, 2 out]
      }
      frame 11 {
        n379 = flat-sequence {
          tunnel: [w1428] -> w1412
          frame #0 {
            w1428 = FALSE ("stop")
            n380 = local write "stop"(w1428) -> ()
          }
        }
        n381 = node-c288() -> (w1427:T1)
        n382 = node-c288() -> (w1425:T1)
        n383 = timed-loop {
          timing: w1427 -> [_]
          timing-out: [_] -> w1426
          tunnel: w1411 -> [w1480]
          tunnel: [w1477] -> w1419
          tunnel: [w1475] -> w1423
          tunnel: [w1474] -> w1422
          tunnel: [w1473] -> w1420
          stop <- TRUE stop-if-true
          n384 = flat-sequence {
            tunnel: w1480 -> [w1482]
            tunnel: [w1482] -> w1478
            tunnel: [w1481] -> w1474
            tunnel: w1478 -> [w1485]
            tunnel: [w1484] -> w1476
            tunnel: [w1483] -> w1472
            tunnel: [w1491] -> w1477
            tunnel: w1476 -> [w1491]
            tunnel: [w1490] -> w1475
            tunnel: [w1489] -> w1473
            tunnel: w1472 -> [w1489]
            frame #0 {
              n385 = call <vilib>:"High Resolution Relative Seconds.vi"() -> ("relative seconds"=w1481:dbl)
            }
            frame #1 {
              w1483 = 10000
              n386 = for {
                N: w1483 -> [_]
                shift-right: [w1486] -> w1484
                shift-left: w1485 -> [w1486]
                shift-right: [w1487] -> _
                shift-left: _ -> [_]
                n387 = local read "local"() -> (w1488:cluster{"Numeric":u64})
                n388 = Unbundle By Name(w1488) -> ("Numeric"=w1487:u64)
              }
            }
            frame #2 {
              n389 = call <vilib>:"High Resolution Relative Seconds.vi"() -> ("relative seconds"=w1490:dbl)
            }
          }
        }
        n390 = timed-loop {
          timing: w1425 -> [_]
          timing-out: [_] -> w1424
          tunnel: w1419 -> [w1440]
          tunnel: [w1438] -> w1413
          tunnel: [w1435] -> w1416
          tunnel: [TRUE] -> w1410
          stop <- TRUE stop-if-true
          n391 = for {
            N: 100000 -> [_]
            shift-right: [w1451] -> w1438
            shift-left: w1440 -> [w1452]
            shift-right: [w1445] -> w1435
            shift-left: 0.0 -> [w1446]
            shift-right: [w1444] -> _
            shift-left: _ -> [w1450]
            i -> [w1442]
            n392 = flat-sequence {
              tunnel: w1452 -> [w1461]
              tunnel: [w1461] -> w1454
              tunnel: [w1460] -> w1448
              tunnel: w1450 -> [w1459]
              tunnel: [w1459] -> w1453
              tunnel: w1454 -> [w1462]
              tunnel: w1453 -> [_]
              tunnel: [w1463] -> w1443
              tunnel: [w1462] -> w1441
              tunnel: [w1467] -> w1451
              tunnel: [w1466] -> w1449
              tunnel: [w1465] -> w1444
              tunnel: w1443 -> [w1465]
              tunnel: w1441 -> [w1467]
              frame #0 {
                n393 = call <vilib>:"High Resolution Relative Seconds.vi"() -> ("relative seconds"=w1460:dbl)
              }
              frame #1 {
                n394 = local read "local"() -> (w1464:cluster{"Numeric":u64})
                n395 = Unbundle By Name(w1464) -> ("Numeric"=w1463:u64)
              }
              frame #2 {
                n396 = call <vilib>:"High Resolution Relative Seconds.vi"() -> ("relative seconds"=w1466:dbl)
              }
            }
            n397 = Subtract(x=w1449, y=w1448) -> (x-y=w1447:dbl)
            n398 = case shown="0" w1442 {
              tunnel: w1447 -> [_ w1458]
              tunnel: w1446 -> [w1455 w1457]
              tunnel: [w1455 w1456] -> w1445
              frame 0 {
              }
              frame 1, Default {
                n399 = Max & Min(x=w1458, y=w1457) -> (max(x,y)=w1456:dbl)  [unwired: 1 out]
              }
            }
          }
        }
        "Max raw local" <- w1416
        n400 = while {
          tunnel: w1412 -> [_]
          tunnel: w1411 -> [_]
          i -> [w1431]
          stop <- "stop" stop-if-true
          n401 = Bundle By Name(cluster=cluster{"Numeric":u64} {"Numeric"=0} ("local"), "Numeric"=w1431) -> (w1433:cluster{"Numeric":u64})
          n402 = local write "local"(w1433) -> ()
          n403 = Wait (ms)(milliseconds to wait=u32 0) -> ()  [unwired: 1 out]
        }
        n404 = node-c288(w1426) -> ()  [unwired: 1 out]
        n405 = node-c288(w1424) -> ()  [unwired: 1 out]
        n406 = Subtract(x=w1423, y=w1422) -> (x-y=w1421:dbl)
        n407 = local write "stop"(w1410) -> ()
        n408 = Divide(x=w1421, y=w1420) -> (x/y=w1418:dbl)
        "avg raw local" <- w1418
        n409 = Less?(x=w1416, y=9e-07) -> (x < y?=w1414:bool)
        n410 = Less?(x=w1418, y=5e-07) -> ()  [unwired: 1 out]
      }
    }
  }
  "error out" <- w4
  n411 = And Array Elements(Boolean array=w2) -> (logical AND=→"pass":bool)
